vi "main.vi"() -> ()   [LabVIEW 2021]
uses:
  daq.ctl
  gpibusb.ctl
  calib.ctl
  <vilib>/Analysis/6fits.llb/Curve Fitting Criteria.ctl
  daq_FSM.vi
  Arduino_FlowPump_Controller.vi
  <vilib>/ErrorRing/Error Ring.xnode
  DAQ.lvlib
  CALIBRATION.lvlib
  statistics.lvlib
  <vilib>/Analysis/NI_AALPro.lvlib
  <vilib>/Analysis/NI_AALBase.lvlib
  GPIB_UART.lvlib
  Certification.lvlib
panel:
  out "Hysteresis Graph":cluster{dbl[], "Media":dbl[]}[](graph)
  out "Uncertainty linearity error":dbl
  out "Hysteresis Uncertainty":dbl
  out "Accuracy Reference Instrument (FS-2012)":dbl
  out "Standard Uncertainty DAQ (mL/min)":dbl
  out "sum of squared errors":dbl
  out "max value":dbl
  out "x/y":dbl
  out "Array":dbl[](array[numeric])
  out "Media 2":dbl[](array[numeric])
  out "Media":dbl[](array[numeric])
  out "Max Uncertainty\n (Descending) [mV]":dbl format="%_1f"
  out "Max Uncertainty\n (Ascending) [mV]":dbl format="%#_2f"
  out "Max Combined \nUncertainty (RSS) [mL/min]\n\n2":dbl format="%_3f"
  out "Max Uncertainty\n (Ascending) [mL/min]\n\n2":dbl format="%_3f"
  out "Max Uncertainty\n (Descending) [mL/min]\n\n2":dbl format="%_3f"
  out "Max Combined \nUncertainty (RSS) [mV]":dbl format="%.1f"
  out "digital_salita_2":dbl[][](array[numeric])
  out "digital_salita_1":dbl[][](array[numeric])
  out "digital_discesa_2":dbl[][](array[numeric])
  out "digital_discesa_1":dbl[][](array[numeric])
  out "analog_salita_2":dbl[][](array[numeric])
  out "analog_salita_1":dbl[][](array[numeric])
  out "analog_discesa_2":dbl[][](array[numeric])
  out "analog_discesa_1":dbl[][](array[numeric])
  out "Max Uncertainty Descending":dbl format="%#.1f"
  out "Max Uncertainty Asending.":dbl format="%#.1f"
  out "abs(x)":dbl[](array[numeric])
  out "difference":dbl[](array[numeric])
  out "asc_table":dbl[][](array[numeric])
  out "disc_table 2":dbl[][](array[numeric])
  out "Estimate Ascending":dbl[](array[numeric])
  out "Estimate Descending":dbl[](array[numeric])
  out "Best Linear Fit D2":dbl[](array[numeric])
  out "Best Linear Fit D":dbl[](array[numeric])
  out "total_flow":dbl[][](array[numeric])
  out "Best Linear Fit A":dbl[](array[numeric])
  out "Standard Uncertainty DAQ (mV)":dbl
  out "eqA":string
  out "eqD":string
  out "Table Strings":string[][](array[string])
  out "step_":i32
  out "start_":i32
  in  "scale_analog":dbl=1000.0
  in  "scale_digital":dbl=1000.0
  out "Input Sequence":dbl[](array[numeric])
  in  "Tab Control":T1(tab)
  in  "Tab Control 7":enum32{"POWER PANEL", "Contacts"}(tab)
  in  "POWER":bool=TRUE
  in  "POWER 2":bool=TRUE
  in  "POWER 3":bool=TRUE
  in  "Base Programs Path":path=path "C:/Users/anton/Desktop/mapi-master"
  out "String":string="Welcome! This is the main application to use in order to calibrate the analog flow sensor, Renesas FS-1012.\n\nThe picture to the left shows the instruments that you will need to connect to use this application. These are:\na) NI DAQ-6008 Data Acquisition Board\nb) Conditioning circuit\nc) Analog (under test) Flow Sensor, Renesas FS-1012\nd) Digital (reference) Flow Sensor, Renesas FS-2012\ne) air-pump\nf) Power Generator Agilent e36436A\ng) Power Supply QL355TP\n\n\nEach Tab in the application allows to perform the many steps that compose the calibration procedure to follow in order to be able to convert the raw output of the sensor (voltage, in mV) into a significant measure (flow, in liters-per-minute). \n\nThe following is a brief description of what each tab enables to accomplish:\n1) Acquisition: this tab enables you to perform acquisitions from both sensors as well as save the acquired samples in specified files.\n2) Datasets: this tab enables you to load the stored dataset to begin the analysis of each sensor.\n3) Visual Exploration: this tab enables you to get a first view of the statistical distribution of the samples in each dataset, through histograms and boxplots.\n4) Results: this tab is used to compare the measurements acquired during ascending and descending input sequences in order to verify the occurrence of the hysteresis phenomena. Also, sensor accuracy is reported in specified indicators.\n5) Comparison: this tab enable the user to compare the plot of ascending and descending curves of both sensors, in order to determine whether the measurements taken from the two instruments share some kind of correlation.\n6) Curve Fitting: this tab enables you to compute the best-fit equations to predict the output value of each sensor given the input current that drives the air-pump, which in turn generates an airflow measured by the two sensors, respectively.\n7) Instruments Control: this tab should be used only be expert users. It enables you to control directly the power generator and the Arduino UNO, through dedicated controls.\n\nReference manuals will explain in more detail the correct way to use this application!"
  in  "Tab Control 8":T2(tab)
  out "FS-2012 ON|OFF 2":bool
  out "POWER_SUPPLY ON|OFF 2":bool
  out "DAQ ON|OFF":bool
  out "FS-1012 ON|OFF":bool
  out "ARDUINO ON|OFF 2":bool
  in  "gpib address":string(combo)="1"
  in  "serial port":string(combo)="COM5"
  in  "Channel":string(combo)="Dev1/ai0"
  in  "Phase":string(combo)="tabella_salita"
  in  "Ring 2":u16(ring)=1 items=["Dataset 1"=1, "Dataset 2"=2]
  in  "Read":bool
  in  "Samples":i32=100
  in  "Control Panel":T3={"Enable"=FALSE, "Step [mA]"=0, "Next"=FALSE, "Start [mA]"=400} {"Start [mA]" min=0 max=1000 step=25; "Step [mA]" min=0 max=1000 step=25}
  out "output current":i32(knob)=400 scale=0.0..700.0
  in  "Dataset A Path":path=path "C:/Users/anton/Desktop/Measurements_stuff/sandbox/last"
  in  "Dataset D Digital":path=path "C:/Users/anton/Desktop/Measurements_stuff/sandbox/last"
  in  "Tab Control 2":enum32{"Live Acquisition", "Datasets"}(tab)
  out "volt":dbl format="%#_3g"
  out "flow":dbl
  in  "Buffer Size (Sa)":string(combo)="1000"
  in  "Sampling Rate (Sa/s)":string(combo)="1000"
  in  "Scale Voltage":string(combo)="(mV)"
  in  "Sampling Frequency (Hz)":string(combo)="1.5"
  in  "Scale Flow":string(combo)="(mL/min)"
  out "Analog  Flow Sensor":dbl[](graph)
  out "Digital  Flow Sensor":dbl[](graph)
  in  "DATASET_CLEAR":bool
  in  "DATASET_STORE":bool
  out "Flow Rate (mL/min)":dbl[](array[numeric])
  out "Voltage (mV)":dbl[](array[numeric]) format="%#_3g"
  out "Analog Dataset":dbl[][](array[numeric]) format="%#_3g"
  out "Digital Dataset":dbl[][](array[numeric]) format="%#.3g"
  in  "Save":bool
  in  "Plot Signals":bool
  out "Features":i32
  out "tot_samples":i32
  in  "Up Button 2":bool
  in  "Up Button":bool
  in  "Analog_salita2":path=path "C:/Users/anton/Desktop/mapi-master/misure_17_10_A/tab_salita2.csv"
  in  "Analog_salita1":path=path "C:/Users/anton/Desktop/mapi-master/misure_17_10_A/tab_salita1.csv"
  in  "Analog_discesa2":path=path "C:/Users/anton/Desktop/mapi-master/misure_17_10_A/tab_discesa2.csv"
  in  "Analog_discesa1":path=path "C:/Users/anton/Desktop/mapi-master/misure_17_10_A/tab_discesa1.csv"
  in  "Digital_discesa2":path=path "C:/Users/anton/Desktop/mapi-master/misure_17_10_D/tab_discesa2.csv"
  in  "Digital_discesa1":path=path "C:/Users/anton/Desktop/mapi-master/misure_17_10_D/tab_discesa1.csv"
  in  "CLEAR BUTTON":bool
  in  "Load Files":bool
  in  "?":enum32{"FS-1012 A", "FS-1012 D"}(tab)
  out "Analog Salita":dbl[][](array[numeric])
  out "Analog Discesa":dbl[][](array[numeric])
  in  "Digital_salita2":path=path "C:/Users/anton/Desktop/mapi-master/misure_17_10_D/tab_salita2.csv"
  in  "Digital_salita1":path=path "C:/Users/anton/Desktop/mapi-master/misure_17_10_D/tab_salita1.csv"
  in  "?":enum32{"FS-2012 D", "FS-2012 A"}(tab)
  out "Digital Discesa":dbl[][](array[numeric])
  out "Digital Salita":dbl[][](array[numeric])
  out "L1":dbl format="%.1f"
  out "U1":dbl format="%.1f"
  in  "index":string(combo)="12" caption="Input Current (mA)"
  in  "Ring":u16(ring)=1 items=["Dataset 2", "Dataset 1"]
  in  "Histogram intervals":i32=10
  in  "Sensor & Phase":T4(ring)=enum."Analog (Decreasing Values)"
  in  "Tab Control 3":enum32{"Histogram", "Boxplot"}(tab)
  out "Histogram":cluster{"X Values":dbl[], dbl[]}[](graph)
  out "Box Plot":cluster{dbl[], dbl[]}[](graph)=[{[7.857142857142858, 2.142857142857143, 2.142857142857143, 7.857142857142858, 7.857142857142858, 2.142857142857143, 2.142857142857143], [0.6526, 0.6526, 0.6514, 0.6514, 0.6538, 0.6538, 0.6526]}, {[], []}, {[5.0, 5.0], [0.6489, 0.6569]}, {[5.0, 5.0], [0.6538, 0.6562000000000001]}, {[5.0, 5.0], [0.6514, 0.6489999999999998]}, {[6.428571428571429, 3.571428571428571], [0.6562000000000001, 0.6562000000000001]}, {[6.428571428571429, 3.571428571428571], [0.6489999999999998, 0.6489999999999998]}, {[17.857142857142858, 12.142857142857142, 12.142857142857142, 17.857142857142858, 17.857142857142858, 12.142857142857142, 12.142857142857142], [0.66495, 0.66495, 0.6635, 0.6635, 0.6662, 0.6662, 0.66495]}, {[15.0, 15.0], [0.6921, 0.6851]}, {[15.0, 15.0, 15.0, 15.0, 15.0, 15.0], [0.6591, 0.6608, 0.6604, 0.6607, 0.671, 0.6606]}, {[15.0, 15.0], [0.6662, 0.669]}, {[15.0, 15.0], [0.6635, 0.6609]}, {[16.428571428571427, 13.571428571428571], [0.669, 0.669]}, {[16.428571428571427, 13.571428571428571], [0.6609, 0.6609]}, {[27.857142857142858, 22.142857142857142, 22.142857142857142, 27.857142857142858, 27.857142857142858, 22.142857142857142, 22.142857142857142], [0.6796, 0.6796, 0.6789, 0.6789, 0.6803, 0.6803, 0.6796]}, {[], []}, {[25.0, 25.0, 25.0, 25.0, 25.0, 25.0, 25.0, 25.0, 25.0], [0.677, 0.6769, 0.6774, 0.6768, 0.6772, 0.6757, 0.6762, 0.6818, 0.6823]}, {[25.0, 25.0], [0.6803, 0.6817000000000001]}, {[25.0, 25.0], [0.6789, 0.6774999999999999]}, {[26.428571428571427, 23.571428571428573], [0.6817000000000001, 0.6817000000000001]}, {[26.428571428571427, 23.571428571428573], [0.6774999999999999, 0.6774999999999999]}]
  out "Q3":dbl format="%.1f"
  out "Q1":dbl format="%.1f"
  out "Mean":dbl format="%.2f"
  out "Standard Deviation":dbl format="%.2f"
  out "Median":dbl format="%.1f"
  in  "Tab Control 6":T5(tab)
  out "Ascending Table":dbl[][](array[numeric]) format="%#.1f"
  out "Descending Table":dbl[][](array[numeric]) format="%#.1f"
  out "uncda":dbl[](array[numeric]) caption="Type A Standard Uncertainties FS-2012 (mL/min)" format="%#.1f"
  out "Standard Deviations FS-1012 (mV)":dbl[](array[numeric]) format="%#_2f"
  out "Standard Deviations FS-2012 (mL/min)":dbl[](array[numeric]) format="%#.1f"
  out "Expected Values FS-1012 (mV)":dbl[](array[numeric]) format="%#.1f"
  out "Expected Values FS-2012 (mL/min)":dbl[](array[numeric]) format="%#.1f"
  out "uncaa":dbl[](array[numeric]) caption="Type A Standard Uncertainties FS-1012 (mV)" format="%#.1g"
  out "uncdd":dbl[](array[numeric]) caption="Type A Standard Uncertainties FS-2012 (mL/min)" format="%#.1f"
  out "uncad":dbl[](array[numeric]) caption="Type A Standard Uncertainties FS-1012 (mV)" format="%#.1f"
  out "stdad":dbl[](array[numeric]) caption="Standard Deviations FS-1012 (mV)" format="%#_2g"
  out "stddd":dbl[](array[numeric]) caption="Standard Deviations FS-2012 (mL/min)" format="%#.1f"
  out "exad":dbl[](array[numeric]) caption="Expected Values FS-1012 (mV)" format="%#.1f"
  out "exdd":dbl[](array[numeric]) caption="Expected Values FS-2012 (mL/min)" format="%#.1f"
  in  "Tab Control 5":T6(tab)
  out "COMPARISON":T7(graph)
  out "FS-1012 Ascending & Descending Curves":T8(graph)
  out "FS-2012 Ascending & Descending Curves":T8(graph)
  in  "Tab Control 9":T9(tab)
  out "A":cluster{"Media":dbl[], "Media":dbl[]}[](graph) caption="FS-1012 Ascending & Descending Curves"
  out "A 2":cluster{"Media":dbl[], dbl[]}[](graph) caption="FS-1012 Ascending & Descending Curves"
  out "D":cluster{"Media":dbl[], "Media":dbl[]}[](graph) caption="FS-1012 Ascending & Descending Curves"
  out "D 2":cluster{"Media":dbl[], dbl[]}[](graph) caption="FS-1012 Ascending & Descending Curves"
  in  "Tab Control 4":enum32{"Regression", "Linearization"}(tab)
  out "RMSE 2":dbl format="%#.1f"
  out "R_sqr":dbl format="%#_3g"
  out "m":dbl format="%#.2f"
  out "b":dbl format="%#.1f"
  out "Calibration Conversion Equation":string="V = m·F + b"
  out "Ascending Table 2":dbl[][](array[numeric]) format="%#.1f"
  out "nonlinearity":dbl format="%#.2f"
  in  "Plot":enum32{"Item 0", "Radio Selection 4"}(radio)=enum."Radio Selection 4"
  out "Calibration Curve":cluster{dbl[], "Media":dbl[]}[](graph)
  in  "Tab Control 10":enum32{"Calibration Curve", "Accuracy"}(tab)
  out "R-square avg":dbl format="%#.2f"
  out "RMSE_avg":dbl format="%#.2f"
  out "b avg":dbl format="%#.1f"
  out "m avg":dbl format="%#.2f"
  out "Calibration Conversion Equation 2":string="V = m·F + b"
  out "Absolute Uncertainty in %FSO":dbl format="%#.2f"
  out "Expanded Uncertainty in %FSO":dbl format="%#.2f"
  out "Nonlinearity %FSO":dbl format="%#.2f"
  out "Hysteresis %FSO":dbl format="%#.2f"
  out "Max Uncertainty":dbl format="%#.1f"
  out "Max Deviation":dbl format="%#.1f"
  out "Absolute Uncertainty":dbl format="%#.1f"
  out "Expanded Uncertainty":dbl format="%#.1f"
  in  "calibrate!":bool
  in  "Arduino":string="Arduino UNO R3"
  in  "Air Pump":string="EAD NEO PP2"
  in  "DAQ":string="NI USB-6008"
  in  "PSU A":string="Agilent, Type e3634A"
  in  "Gas used":string="Air"
  in  "DAQ Resolution":string="4,88"
  in  "Location":string="PalaUnisannio"
  in  "Manufacturer":string="Renesas Electronic Company"
  in  "Operator":string="User1"
  in  "Date":string="28/07/2025"
  in  "Temperature":string="25°C"
  in  "Sensing Range":string="0 -10 L/m"
  in  "Series":string="FS-1012-1100-NG"
  in  "Description":string="Gas Flow Meter"
  # "Max Uncertainty\nAscending"
  # "(mL/min)"
  # "(mL/min)"
  # "Max Uncertainty\nDescending"
  # "(mL/min)"
  # "Offset"
  # "Max [mL/min]"
  # "QUICK GUIDE"
  # "DAQ"
  # "MAIN"
  # "GPIB_USB"
  # "mapiflowproject@gmail.com"
  # "programmable power generator"
  # "NI DAQ\nUSB-6008"
  # "ArduinoUNO"
  # "Air-pump"
  # "external \n  power \n  generator"
  # "FS-2012"
  # "FS-1012"
  # "conditioning_circuit"
  # "MEASUREMENT SYSTEM SETUP"
  # "ARDUINO & POWER SUPPLY"
  # "NI-DAQ USB 6008"
  # "ACQUISITION"
  # "Control Panel"
  # "Air Pump\nCurrent [mA]"
  # "FS-2012"
  # "Flow"
  # "FS-1012"
  # "Voltage"
  # "FS-1012"
  # "FS-2012"
  # "D"
  # "A"
  # "DATASETS"
  # "FS-1012"
  # "FS-2012"
  # "Descending Phase"
  # "Descending Phase"
  # "DATASET 1"
  # "DATASET 1"
  # "DATASET 2"
  # "DATASET 2"
  # "Ascending Phase"
  # "DATASET 1"
  # "DATASET 2"
  # "Features Found"
  # "Total No. of Samples"
  # "Analog Sensor Files Here!"
  # "Digital Sensor Files Here!"
  # "(mV)"
  # "Ascending Phase"
  # "(mV)"
  # "Descending Phase"
  # "Ascending Phase"
  # "DATASET 1"
  # "DATASET 2"
  # "(mL/min)"
  # "Descending Phase"
  # "Descending Phase"
  # "(mL/min)"
  # "Ascending Phase"
  # "SETTINGS"
  # "HISTOGRAM"
  # "Mean"
  # "Standard Deviation"
  # "BOXPLOT"
  # "Lower Whisker"
  # "Lower Quartile"
  # "Upper Whisker"
  # "Upper Quartile"
  # "Median"
  # "VISUALIZE"
  # "RESULTS"
  # "Ascending Phase"
  # "FS-1012 (mV)                     | FS-2012 (mL/min)"
  # "Descending Phase"
  # "FS-1012 (mV)                    | FS-2012 (mL/min)"
  # "Comparison Graph"
  # "Ascending Phase Curve"
  # "Descending Phase Curve"
  # "BEST LINEAR FIT"
  # "LINEAR REGRESSION Curve"
  # "Estimated Flow vs. Calibrated Reference"
  # "LINEAR REGRESSION Curve"
  # "Estimated Flow vs. Calibrated Reference"
  # "("
  # ")"
  # "mV"
  # "m"
  # "________"
  # "(mV)"
  # "RMSE"
  # "mL/min"
  # "b"
  # "2"
  # "R"
  # "(mV)"
  # "Linear Regression Equation"
  # "Nonlinearity (%FSO)"
  # "Reference [mL/min]    | DUT       [mL/min]     | Deviation [mL/min]"
  # "Calibration Curve"
  # "Calibration Function f(F)"
  # "("
  # ")"
  # "mV"
  # "m"
  # "b"
  # "________"
  # "(mV)"
  # "mL/min"
  # "2"
  # "R"
  # "RMSE (mV)"
  # "Max. Deviation\n(Asc. vs. Desc.)"
  # "(mL/min)"
  # "Hysteresis"
  # "(%FSO)"
  # "Ascending, Descending Phase\nCombined  Uncertainty (RSS)"
  # "Nonlinearity"
  # "(%FSO)"
  # "(mL/min)"
  # "Measuring System \nAbsolute Uncertainty (%FSO)"
  # "Measuring System \nCombined Uncertainty (mL/min)"
  # "Expanded  Absolute Uncertainty, k = 2  (%FSO)"
  # "Expanded  Combined Uncertainty, k = 2  (mL/min)"
  # "Manufacturer"
  # "Description"
  # "Gas Used"
  # "PSU"
  # "Sensing Range (Nominal)"
  # "Series"
  # "DAQ Resolution (mV)"
  # "DAQ"
  # "Flow Pump"
  # "Arduino"
  # "Environment Temperature"
  # "Date"
  # "Operator"
  # "Location"
  # "Instrumentation Used"
  # "General Informations"
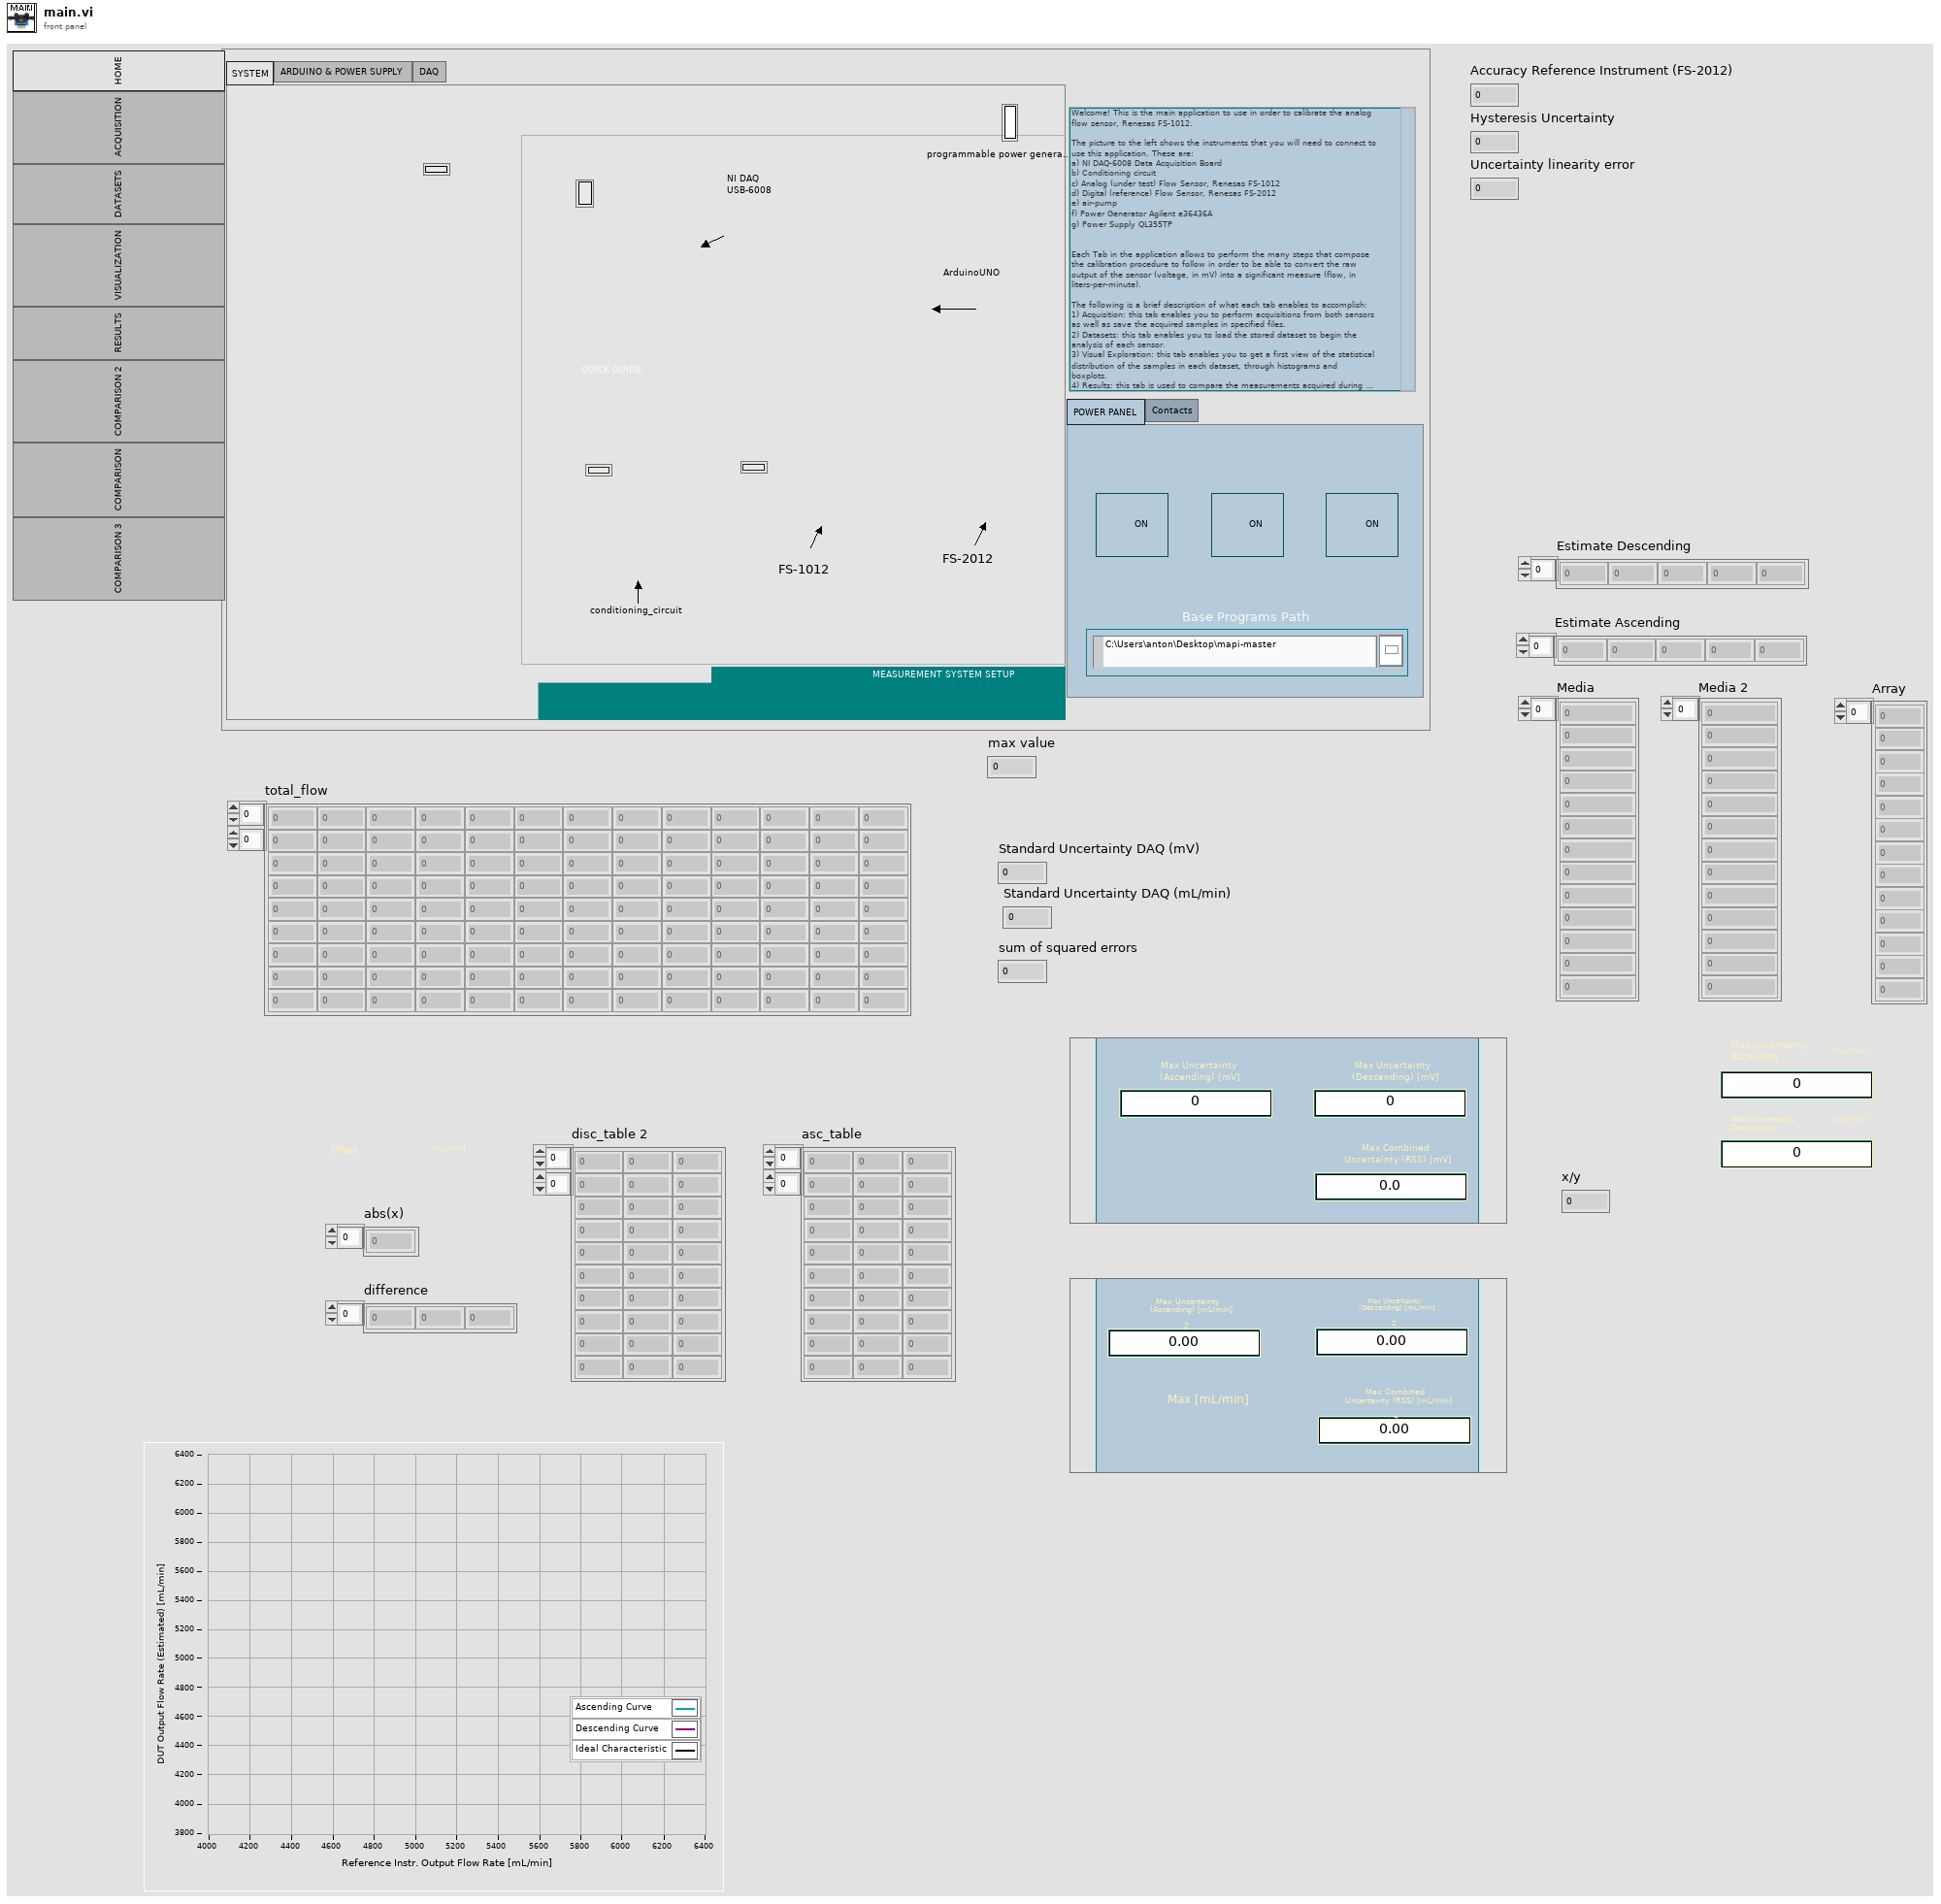
[diagram p1: front panel]
types:
  T1 = enum32{"HOME", "ACQUISITION", "DATASETS", "VISUALIZATION", "RESULTS", "COMPARISON 2", "COMPARISON", "COMPARISON 3"}
  T2 = enum32{"SYSTEM", "ARDUINO & POWER SUPPLY", "DAQ"}
  T3 = cluster{"Enable":bool, "Step [mA]":i32, "Next":bool, "Start [mA]":i32}
  T4 = enum16{"Analog (Increasing Values)", "Analog (Decreasing Values)", "Digital (Decreasing Values)", "Digital (Increasing Values)"}
  T5 = enum32{"Comparison Tables", "Analysis (A)", "Analysis (D)"}
  T6 = enum32{"Comparison", " Ascending", " Descending"}
  T7 = cluster{"Array":dbl[], "media_combinata":dbl[]}[]
  T8 = cluster{"media_combinata":dbl[], "Array":dbl[]}[]
  T9 = enum32{"Ascending (Voltage vs. Flow)", "Ascending (Flow in vs. Flow Out)", "Descending (Voltage vs. Flow)", "Descending (Flow in vs. Flow out)"}
  T10 = typedef "calib.ctl" = enum16{"wait", "linearization", "certificate", "linear regression", "simulate", "results4", "result3", "curves", "fitting", "results2", "combined uncertainty", "results", "boxplot", "scatterplot", "comparison", "histogram", "error", "curve_fitting", "calibration curve", "uncertainty", "load_measures", ""}
  T11 = typedef "gpibusb.ctl" = enum16{"INIT", "FREQ", "CURR?", "CURR", "READ_DIGITAL", "START", "STOP", "ACQUIRE", "STEP", "ARDUINO_SETTINGS", "NEXT", "SHUTDOWN", "ERROR"}
  T12 = typedef "daq.ctl" = enum16{"INIT", "PARAMETERS", "READ", "READ_VOLTAGE", "STOP", "DAQ_SETTINGS", "ERROR", "FLUSH", "SHUTDOWN", "CLEAR"}
  T13 = enum8{"Enabled", "Disabled", "Disabled and Grayed Out"}
  T14 = cluster{"Description":string, "Manufacturer":string, "Series":string, "Sensing Range":string, "Operator":string, "Temperature":string, "PSU A":string, "PSU B":string, "Gas used":string, "Air Pump":string, "DAQ":string, "Arduino":string}
  T15 = typedef "NI_AALPro.lvlib/Curve Fitting Criteria.ctl" = u16
  T16 = cluster{"Media":dbl[], "Best Linear Fit":dbl[]}[]
  T17 = cluster{"Media":dbl[], "Estimate Descending":dbl[]}
  T18 = cluster{"Media":dbl[], "Estimate Ascending":dbl[]}
  T19 = cluster{"Media":dbl[], "Estimate Ascending":dbl[]}[]
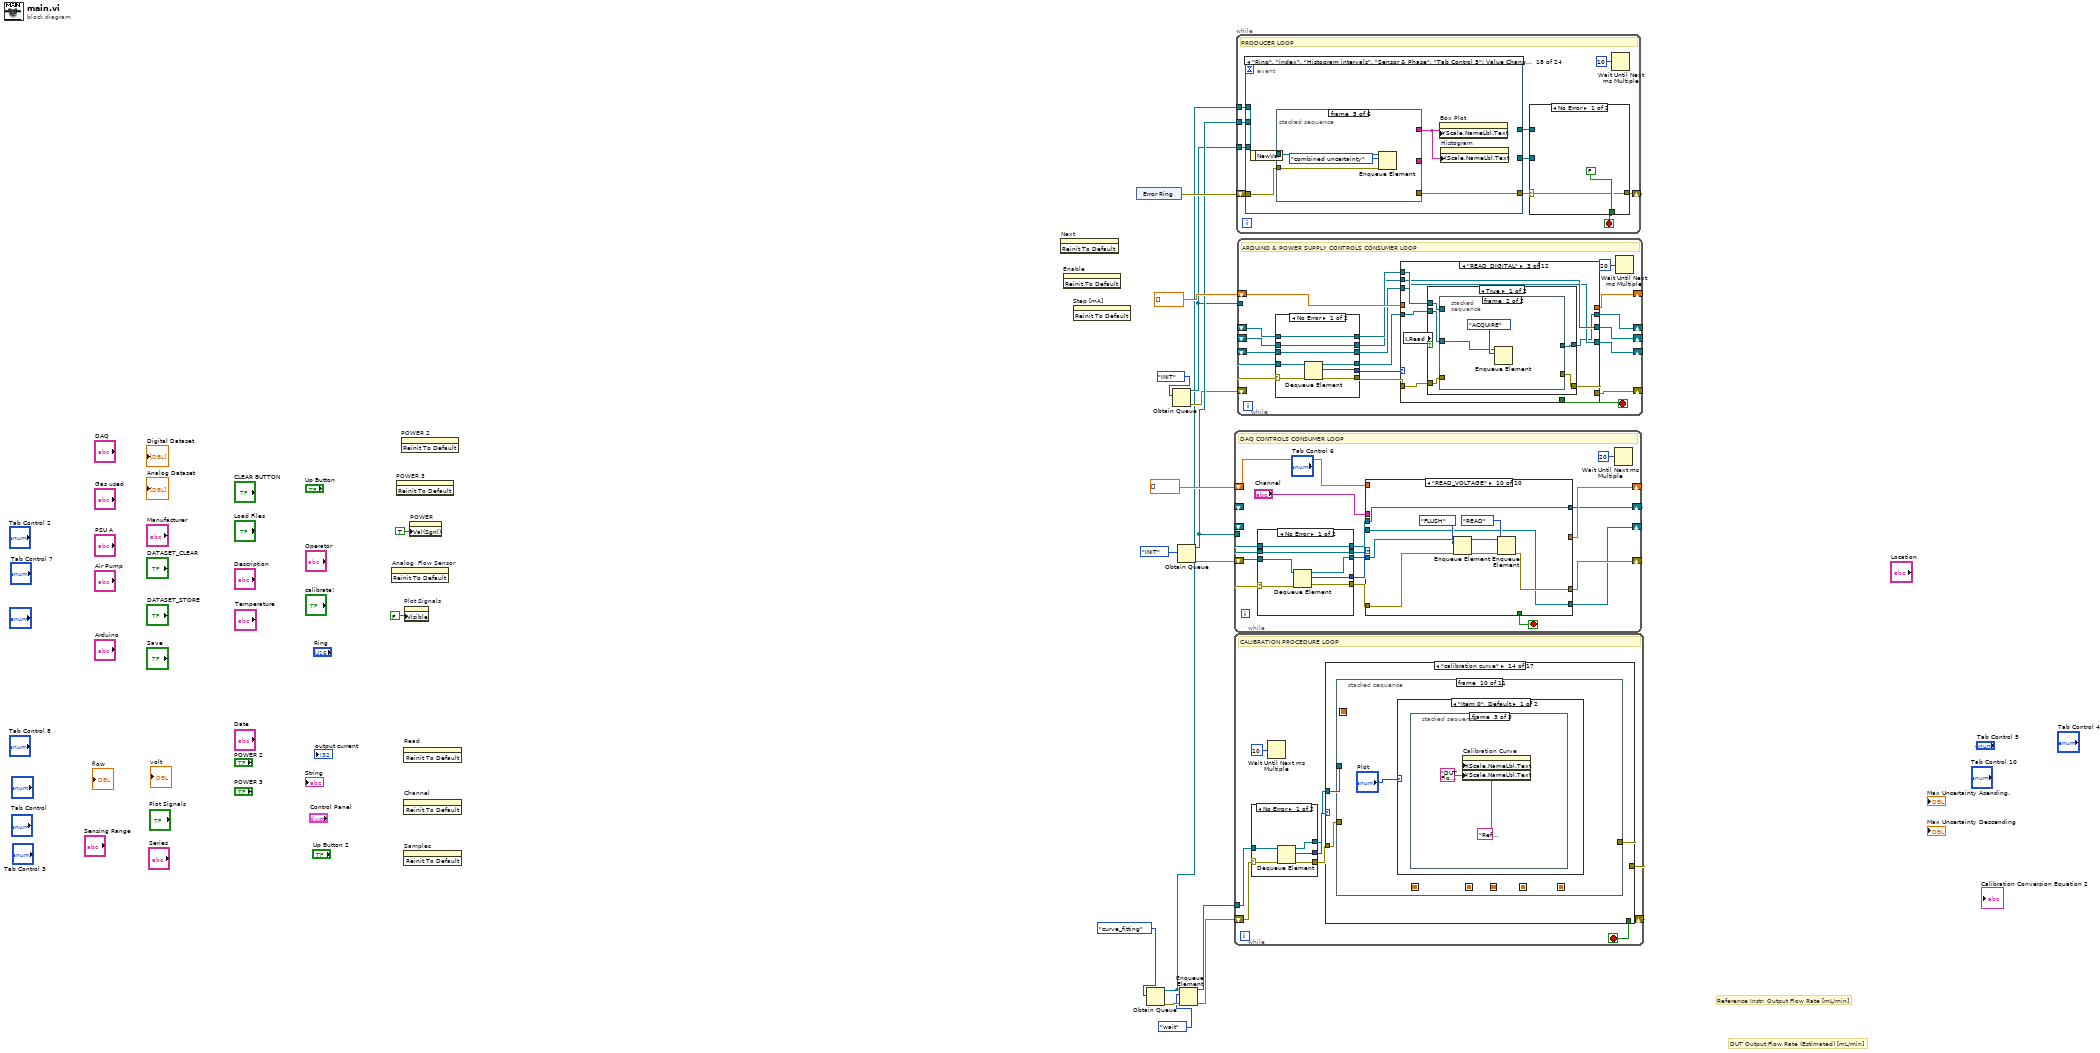
[diagram p0: block diagram]
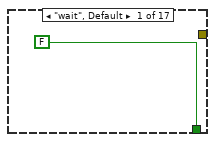
[diagram p2: hidden frame]
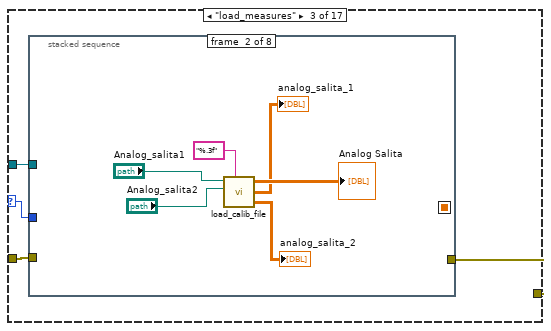
[diagram p4: hidden frame]
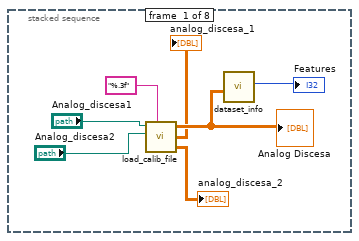
[diagram p5: hidden frame]
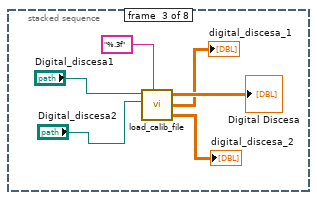
[diagram p6: hidden frame]
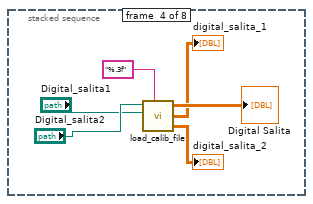
[diagram p7: hidden frame]
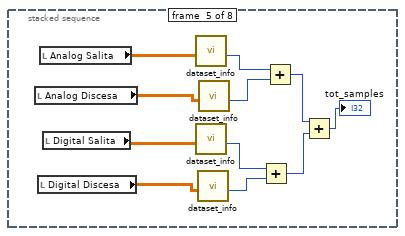
[diagram p8: hidden frame]
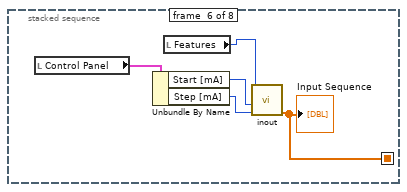
[diagram p9: hidden frame]
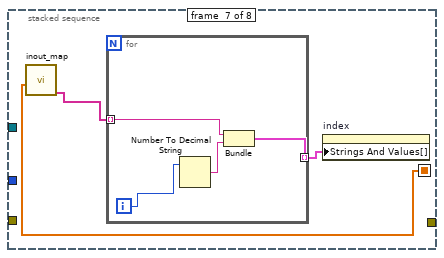
[diagram p10: hidden frame]
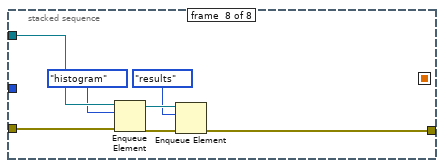
[diagram p11: hidden frame]
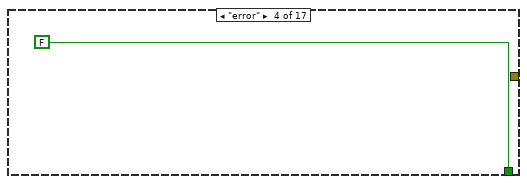
[diagram p12: hidden frame]
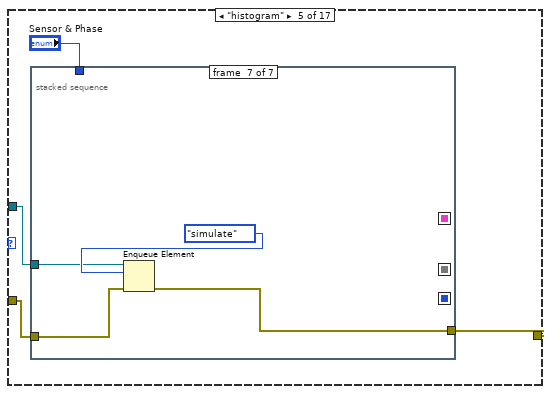
[diagram p13: hidden frame]
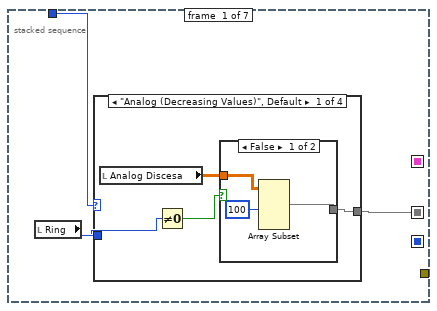
[diagram p14: hidden frame]
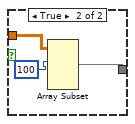
[diagram p15: hidden frame]
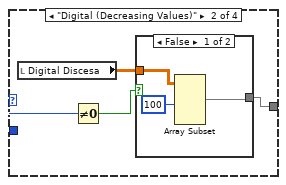
[diagram p16: hidden frame]
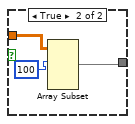
[diagram p17: hidden frame]
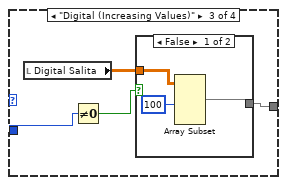
[diagram p18: hidden frame]
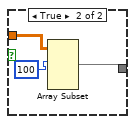
[diagram p19: hidden frame]
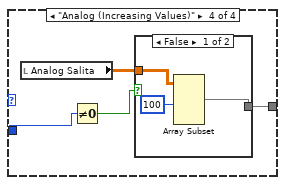
[diagram p20: hidden frame]
diagram:
  # "DUT Output Flow Rate (Estimated) [mL/min]"
  # "Reference Instr. Output Flow Rate [mL/min]"
  n1 = invoke on="Analog  Flow Sensor" class="WFGraph (strict)" method="Reinit To Default"() -> ()  [unwired: 3 in, 3 out]
  n2 = invoke on="POWER 3" class="Bool (strict)" method="Reinit To Default"() -> ()  [unwired: 3 in, 3 out]
  n3 = invoke on="POWER 2" class="Bool (strict)" method="Reinit To Default"() -> ()  [unwired: 3 in, 3 out]
  n4 = invoke on="Read" class="Bool (strict)" method="Reinit To Default"() -> ()  [unwired: 3 in, 3 out]
  n5 = invoke on="Channel" class="CmbBox" method="Reinit To Default"() -> ()  [unwired: 3 in, 3 out]
  n6 = invoke on="Samples" class="DigNum (strict)" method="Reinit To Default"() -> ()  [unwired: 3 in, 3 out]
  n7 = property on="Plot Signals" class="Bool"("Visible"=FALSE) -> ()  [unwired: 2 in, 2 out]
  n8 = property on="POWER" class="Bool (strict)"("Val(Sgnl)"=TRUE ("Value (Signaling)")) -> ()  [unwired: 2 in, 2 out]
  n9 = invoke on="Next" class="Bool (strict)" method="Reinit To Default"() -> ()  [unwired: 3 in, 3 out]
  n10 = invoke on="Enable" class="Bool (strict)" method="Reinit To Default"() -> ()  [unwired: 3 in, 3 out]
  n11 = invoke on="Step [mA]" class="DigNum (strict)" method="Reinit To Default"() -> ()  [unwired: 3 in, 3 out]
  n12 = xnode "Error Ring"() -> ("error out"=w14:errorcluster)
  n13 = Obtain Queue(element data type=calib."curve_fitting" ("Enum")) -> (queue out=w2:refnum<queue>, error out=w6:errorcluster)  [unwired: 4 in, 1 out]
  n14 = Obtain Queue(element data type=gpibusb."INIT" ("element")) -> (queue out=w10:refnum<queue>, error out=w9:errorcluster)  [unwired: 4 in, 1 out]
  n15 = Obtain Queue(element data type=daq."INIT" ("STATE")) -> (queue out=w11:refnum<queue>, error out=w8:errorcluster)  [unwired: 4 in, 1 out]
  n16 = Enqueue Element(queue=w2, element=calib."wait", error in (no error)=w6) -> (queue out=w4:refnum<queue>, error out=w5:errorcluster)  [unwired: 1 in, 1 out]
  n17 = while {
    tunnel: w11 -> [w33]
    shift-right: [w27] -> _
    shift-left: dbl[] [] -> [w28]
    shift-right: [w26] -> _
    shift-left: w8 -> [w34]
    shift-right: [w24] -> _
    shift-left: _ -> [w22]
    shift-right: [w23] -> _
    shift-left: _ -> [w21]
    stop <- w29 stop-if-true
    # "DAQ CONTROLS CONSUMER LOOP"
    n18 = case shown="No Error" w34 {
      selector: w34 -> [w40 w46]
      tunnel: w33 -> [w41 w44]
      tunnel: [w39 daq."ERROR" ("STATE")] -> w32
      tunnel: [w38 w46] -> w31
      tunnel: [w37 w44] -> w30
      tunnel: [w36 w43] -> w19
      tunnel: w22 -> [w36 w43]
      tunnel: [w35 w42] -> w20
      tunnel: w21 -> [w35 w42]
      frame No Error {
        n19 = Dequeue Element(queue=w41, error in (no error)=w40) -> (queue out=w37:refnum<queue>, element=w39:T12, error out=w38:errorcluster)  [unwired: 1 in, 1 out]
      }
      frame Error {
      }
    }
    n20 = case shown="\"READ_VOLTAGE\"" w32 {
      tunnel: w31 -> [w51 w56 w88 w129 w136 w139 w156 w162 w169 w177]
      tunnel: w30 -> [w52 _ w87 _ _ _ _ _ _ w181]
      tunnel: [FALSE FALSE _ _ _ _ _ _ _ _] -> w29
      tunnel: w28 -> [_ _ w90 _ _ _ _ _ _ _]
      tunnel: [_ _ w85 _ _ _ _ _ _ _] -> w27
      tunnel: [w49 w55 w86 w128 _ _ _ w166 w168 w175] -> w26
      tunnel: "Channel" -> [_ _ _ _ w134 _ _ _ _ _]
      tunnel: [w48 w54 w91 w125 w131 w138 w159 w164 w172 w174] -> w24
      tunnel: [w47 w53 w84 w126 w130 w137 w158 w165 w171 w173] -> w23
      tunnel: w20 -> [w47 _ w89 w127 w130 w137 w158 w165 w171 w173]
      tunnel: w19 -> [w48 _ w91 w125 w132 w140 w159 w163 w172 w174]
      frame "ERROR" {
        n21 = Release Queue(queue=w52, error in (no error)=w51) -> (error out=w49:errorcluster)  [unwired: 1 in, 2 out]
      }
      frame "INIT", Default {
        n22 = local read "Base Programs Path"() -> (w57:path)
        n23 = stacked-sequence {
          seq-local: [w61 _ _ _ _ _ _ _ _] -> [_ _ _ _ w73 _ _ _ _]
          seq-local: [_ w64 _ _ _ _ _ _ _] -> [_ _ _ _ _ w76 _ _ _]
          seq-local: [_ _ w66 _ _ _ _ _ _] -> [_ _ _ _ _ w75 _ _ _]
          seq-local: [_ _ _ _ w72 _ _ _ _] -> [_ _ _ _ _ w80 w82 _ _]
          seq-local: [_ _ _ _ w69 _ _ _ _] -> [_ _ _ _ _ w79 _ _ _]
          seq-local: [_ _ _ _ _ w78 _ _ _] -> [_ _ _ _ _ _ _ _ _]
          tunnel: w56 -> [_ _ _ _ w71 _ w81 _ _]
          tunnel: w57 -> [w59 _ _ _ _ _ _ _ _]
          tunnel: [_ _ _ _ _ w76 _ _ _] -> w53
          tunnel: [_ _ _ _ _ _ w83 _ _] -> w55
          tunnel: [_ _ _ _ _ w75 _ _ _] -> w54
          frame #0 {
            # "compose program path"
            n24 = Path To String(path=w59) -> (string=w63:string)
            n25 = Concatenate Strings(w63, "\\labview\\daq_FSM.vi" ("string")) -> (w62:string)
            n26 = String To Path(string=w62) -> (path=w61:path)
          }
          frame #1 {
            n27 = Obtain Queue(element data type="") -> (queue out=w64:refnum<queue>)  [unwired: 4 in, 2 out]
          }
          frame #2 {
            n28 = Obtain Queue(element data type="") -> (queue out=w66:refnum<queue>)  [unwired: 4 in, 2 out]
          }
          frame #3 {
            w68 = TRUE ("Boolean 2")
            "DAQ ON|OFF" <- w68
            "FS-1012 ON|OFF" <- w68
          }
          frame #4 {
            n29 = vi-ref "DAQ.lvlib:daq_FSM.vi"() -> (w70:refnum<vi>)
            n30 = Open VI Reference(type specifier VI Refnum (for type only)=w70, vi path=w73, options=128, error in (no error)=w71) -> (vi reference=w72:refnum<vi>, error out=w69:errorcluster)  [unwired: 2 in]
          }
          frame #5 {
            n31 = call-by-ref "Start Asynchronous Call"(reference=w80, error in=w79, "loop rate"=u32 1000, "commands"=w75, "measurements"=w76) -> (error out=w78:errorcluster)  [unwired: 9 in, 1 out]
          }
          frame #6 {
            n32 = invoke on="DAQ CONTROL PANEL" class="SubPnl" method="Insert VI"(error in=w81, "VI Ref"=w82) -> (error out=w83:errorcluster)  [unwired: 2 in, 3 out]
          }
          frame #7 {
          }
          frame #8 {
          }
        }
      }
      frame "READ" {
        n33 = stacked-sequence {
          seq-local: [w97 _ _] -> [_ w102 w103]
          tunnel: w90 -> [w101 _ _]
          tunnel: w89 -> [w99 _ _]
          tunnel: w88 -> [w98 _ w105]
          tunnel: w87 -> [_ _ w106]
          tunnel: [_ w102 _] -> w85
          tunnel: [_ _ w104] -> w86
          tunnel: [w95 _ _] -> w84
          frame #0 {
            # "FETCH"
            n34 = Dequeue Element(queue=w99, error in (no error)=w98) -> (queue out=w95:refnum<queue>, element=w100:string)  [unwired: 1 in, 2 out]
            n35 = Fract/Exp String To Number(use system decimal point (T)=TRUE, string=w100) -> (number=w93:dbl)  [unwired: 2 in, 1 out]
            n36 = Multiply(x=w93, y="scale_analog") -> (x*y=w92:dbl)
            n37 = Build Array (concatenate)(w101, w92) -> (w97:dbl[])
            n38 = local write "volt"(w92) -> ()
          }
          frame #1 {
            # "update indicators"
            "Analog  Flow Sensor" <- w102
            "Voltage (mV)" <- w102
          }
          frame #2 {
            n39 = local read "Read"() -> (w107:bool)
            n40 = case shown="True" w107 {
              tunnel: w106 -> [_ w112]
              tunnel: [w108 w111] -> w104
              tunnel: w105 -> [w108 w110]
              tunnel: w103 -> [_ w109]
              frame False {
              }
              frame True {
                n41 = stacked-sequence {
                  seq-local: [w114 _ _] -> [_ w120 _]
                  seq-local: [_ w117 _] -> [_ _ w124]
                  tunnel: w112 -> [_ _ w123]
                  tunnel: [_ _ w122] -> w111
                  tunnel: w110 -> [_ _ w121]
                  tunnel: w109 -> [w113 _ _]
                  frame #0 {
                    n42 = Array Size(array=w113) -> (size(s)=w116:i32)
                    n43 = Greater Or Equal?(x=w116, y="Samples") -> (x >= y?=w114:bool)
                  }
                  frame #1 {
                    n44 = Select(t=daq."STOP" ("element"), s=w120, f=daq."READ") -> (s? t:f=w117:T12)
                  }
                  frame #2 {
                    n45 = Enqueue Element(queue=w123, element=w124, error in (no error)=w121) -> (error out=w122:errorcluster)  [unwired: 1 in, 2 out]
                  }
                }
              }
            }
          }
        }
      }
      frame "FLUSH" {
        n46 = Flush Queue(queue=w127, error in (no error)=w129) -> (queue out=w126:refnum<queue>, error out=w128:errorcluster)  [unwired: 1 out]
      }
      frame "DAQ_SETTINGS" {
        n47 = call "conc_state_args.vi"("State"="CONF_CH", "Args"=w134) -> ("state_and_args"=w133:string)  [unwired: 13 in]
        n48 = Enqueue Element(queue=w132, element=w133, error in (no error)=w136) -> (queue out=w131:refnum<queue>)  [unwired: 1 in, 2 out]
      }
      frame "PARAMETERS" {
        n49 = stacked-sequence {
          seq-local: [w143 _] -> [_ w151]
          seq-local: [w142 _] -> [_ w149]
          tunnel: w140 -> [w144 _]
          tunnel: [_ w150] -> w138
          tunnel: [_ w148] -> _
          tunnel: w139 -> [w141 _]
          frame #0 {
            n50 = call "conc_state_args.vi"("State"="CONF:PHY", "Args"="Sampling Rate (Sa/s)") -> ("state_and_args"=w145:string)  [unwired: 13 in]
            n51 = Enqueue Element At Opposite End(queue=w144, element=w145, error in (no error)=w141) -> (queue out=w143:refnum<queue>, error out=w142:errorcluster)  [unwired: 1 in, 1 out]
          }
          frame #1 {
            n52 = call "conc_state_args.vi"("State"="CONF:SAMPLES", "Args"="Buffer Size (Sa)") -> ("state_and_args"=w152:string)  [unwired: 13 in]
            n53 = Enqueue Element At Opposite End(queue=w151, element=w152, error in (no error)=w149) -> (queue out=w150:refnum<queue>, error out=w148:errorcluster)  [unwired: 1 in, 1 out]
          }
        }
      }
      frame "STOP" {
        n54 = property on="Read" class="Bool (strict)"(error in=w156, "Val(Sgnl)"=FALSE ("Value (Signaling)")) -> (error out=w155:errorcluster)  [unwired: 1 in, 1 out]
        n55 = property on="Samples" class="DigNum (strict)"(error in=w155, "DisabledEnum"=T13."Enabled" ("Disabled")) -> ()  [unwired: 1 in, 2 out]
      }
      frame "SHUTDOWN" {
        w161 = FALSE ("DAQ ON|OFF")
        n56 = local write "FS-1012 ON|OFF"(w161) -> ()
        n57 = local write "DAQ ON|OFF"(w161) -> ()
        n58 = Enqueue Element(queue=w163, element="SHUTDOWN", error in (no error)=w162) -> (queue out=w164:refnum<queue>, error out=w166:errorcluster)  [unwired: 1 in, 1 out]
      }
      frame "CLEAR" {
        n59 = property on="Samples" class="DigNum (strict)"(error in=w169, "DisabledEnum"=T13."Enabled" ("Disabled")) -> (error out=w168:errorcluster)  [unwired: 1 in, 1 out]
      }
      frame "READ_VOLTAGE" {
        n60 = Enqueue Element(queue=w181, element=daq."FLUSH", error in (no error)=w177) -> (queue out=w179:refnum<queue>, error out=w178:errorcluster)  [unwired: 1 in, 1 out]
        n61 = Enqueue Element(queue=w179, element=daq."READ", error in (no error)=w178) -> (error out=w175:errorcluster)  [unwired: 1 in, 2 out]
      }
    }
    n62 = Wait Until Next ms Multiple(millisecond multiple=u32 20) -> ()  [unwired: 1 out]
  }
  n63 = while {
    tunnel: w4 -> [w188]
    shift-right: [w182] -> _
    shift-left: w5 -> [w189]
    stop <- w186 stop-if-true
    # "CALIBRATION PROCEDURE LOOP"
    n64 = case shown="No Error" w189 {
      selector: w189 -> [w907 w910]
      tunnel: [w908 w910] -> w183
      tunnel: w188 -> [w906 w909]
      tunnel: [w905 calib."error" ("element")] -> w187
      tunnel: [w904 w909] -> w185
      frame No Error {
        n65 = Dequeue Element(queue=w906, error in (no error)=w907) -> (queue out=w904:refnum<queue>, element=w905:T10, error out=w908:errorcluster)  [unwired: 1 in, 1 out]
      }
      frame Error {
      }
    }
    n66 = Wait Until Next ms Multiple(millisecond multiple=u32 10) -> ()  [unwired: 1 out]
    n67 = case shown="\"calibration curve\"" w187 {
      selector: w187 -> [_ _ w193 _ _ _ _ _ _ _ _ _ _ _ _ _ _]
      tunnel: [FALSE _ _ FALSE _ _ _ _ _ _ _ _ _ _ _ _ _] -> w186
      tunnel: w185 -> [_ _ w194 _ w253 w337 w374 w380 w411 _ w432 w460 w534 w611 _ _ _]
      tunnel: w183 -> [_ _ w192 _ w254 w336 w373 w379 w410 _ w431 w459 w533 w610 _ _ _]
      tunnel: [_ _ w191 _ w251 w335 w371 w378 w409 _ _ w458 w532 w609 _ _ _] -> w182
      frame "wait", Default {
      }
      frame "boxplot" {
      }
      frame "load_measures" {
        n68 = stacked-sequence {
          seq-local: [_ _ _ _ _ w231 _ _] -> [_ _ _ _ _ _ w236 _]
          tunnel: w194 -> [_ _ _ _ _ _ _ w249]
          tunnel: w193 -> [_ _ _ _ _ _ _ _]
          tunnel: w192 -> [_ _ _ _ _ _ _ w247]
          tunnel: [_ _ _ _ _ _ _ w243] -> w191
          frame #0 {
            n69 = call "load_calib_file.vi"("file_1"="Analog_discesa1", "file_2"="Analog_discesa2", "format (%.3f)"="%.3f") -> ("insieme"=w197:dbl[][], "dataset1"=→"analog_discesa_1":dbl[][], "dataset2"=→"analog_discesa_2":dbl[][])  [unwired: 2 in]
            "Analog Discesa" <- w197
            n70 = call "dataset_info.vi"("Analog Salita"=w197) -> ("features"=→"Features":i32)  [unwired: 7 in, 3 out]
          }
          frame #1 {
            n71 = call "load_calib_file.vi"("file_1"="Analog_salita1", "file_2"="Analog_salita2", "format (%.3f)"="%.3f") -> ("insieme"=→"Analog Salita":dbl[][], "dataset1"=→"analog_salita_1":dbl[][], "dataset2"=→"analog_salita_2":dbl[][])  [unwired: 2 in]
          }
          frame #2 {
            n72 = call "load_calib_file.vi"("file_1"="Digital_discesa1", "file_2"="Digital_discesa2", "format (%.3f)"="%.3f") -> ("insieme"=→"Digital Discesa":dbl[][], "dataset1"=→"digital_discesa_1":dbl[][], "dataset2"=→"digital_discesa_2":dbl[][])  [unwired: 2 in]
          }
          frame #3 {
            n73 = call "load_calib_file.vi"("file_1"="Digital_salita2", "file_2"="Digital_salita1", "format (%.3f)"="%.3f") -> ("insieme"=→"Digital Salita":dbl[][], "dataset1"=→"digital_salita_1":dbl[][], "dataset2"=→"digital_salita_2":dbl[][])  [unwired: 2 in]
          }
          frame #4 {
            n74 = local read "Analog Discesa"() -> (w229:dbl[][])
            n75 = local read "Digital Discesa"() -> (w227:dbl[][])
            n76 = local read "Analog Salita"() -> (w230:dbl[][])
            n77 = local read "Digital Salita"() -> (w228:dbl[][])
            n78 = call "dataset_info.vi"("Analog Salita"=w230) -> ("samples"=w226:i32)  [unwired: 7 in, 3 out]
            n79 = call "dataset_info.vi"("Analog Salita"=w228) -> ("samples"=w224:i32)  [unwired: 7 in, 3 out]
            n80 = call "dataset_info.vi"("Analog Salita"=w227) -> ("samples"=w223:i32)  [unwired: 7 in, 3 out]
            n81 = call "dataset_info.vi"("Analog Salita"=w229) -> ("samples"=w225:i32)  [unwired: 7 in, 3 out]
            n82 = Add(x=w224, y=w223) -> (x+y=w221:i32)
            n83 = Add(x=w226, y=w225) -> (x+y=w222:i32)
            n84 = Add(x=w222, y=w221) -> (x+y=→"tot_samples":i32)
          }
          frame #5 {
            n85 = local read "Control Panel"() -> (w233:T3)
            n86 = Unbundle By Name(w233) -> ("Start [mA]"=w235:i32, "Step [mA]"=w234:i32)
            n87 = local read "Features"() -> (w232:i32)
            n88 = call "inout.vi"("Step [mA]"=w234, "Initial Value [mA]"=w235, "# Steps"=w232) -> ("Array"=w231:dbl[])  [unwired: 8 in]
            "Input Sequence" <- w231
          }
          frame #6 {
            n89 = call "inout_map.vi"("Input Sequence"=w236) -> ("array"=w237:string[])  [unwired: 10 in]
            n90 = for {
              tunnel: w237 -> [w242] mode=indexing
              tunnel: [w239] -> w238 mode=indexing
              i -> [w241]
              n91 = Number To Decimal String(number=w241) -> (decimal integer string=w240:string)  [unwired: 1 in]
              n92 = Bundle("format string"=w242, w240) -> (w239:cluster{"format string":string, string})  [unwired: 1 in]
            }
            n93 = property on="index" class="CmbBox"("Strings And Values[]"=w238) -> ()  [unwired: 2 in, 2 out]
          }
          frame #7 {
            n94 = Enqueue Element(queue=w249, element=calib."histogram", error in (no error)=w247) -> (queue out=w246:refnum<queue>, error out=w245:errorcluster)  [unwired: 1 in, 1 out]
            n95 = Enqueue Element(queue=w246, element=calib."results", error in (no error)=w245) -> (error out=w243:errorcluster)  [unwired: 1 in, 2 out]
          }
        }
      }
      frame "error" {
      }
      frame "histogram" {
        n96 = stacked-sequence {
          seq-local: [w256 _ _ _ _ _ _] -> [_ w299 _ w312 w316 w324 _]
          seq-local: [_ w298 _ _ _ _ _] -> [_ _ w305 _ _ _ _]
          seq-local: [_ _ w303 _ _ _ _] -> [_ _ _ w311 w315 w323 _]
          tunnel: "Sensor & Phase" -> [w255 _ _ _ _ _ _]
          tunnel: w254 -> [_ _ _ _ _ _ w333]
          tunnel: [_ _ _ _ _ _ w332] -> w251
          tunnel: w253 -> [_ _ _ _ _ _ w331]
          frame #0 {
            n97 = local read "Ring"() -> (w257:u16)
            n98 = case shown="\"Analog (Decreasing Values)\", Default" w255 {
              tunnel: [w258 w268 w278 w288] -> w256
              tunnel: w257 -> [w259 w269 w279 w289]
              frame "Analog (Decreasing Values)", Default {
                n99 = local read "Analog Discesa"() -> (w260:dbl[][])
                n100 = Not Equal To 0?(x=w259) -> (x != 0?=w261:bool)
                n101 = case shown="False" w261 {
                  tunnel: w260 -> [w264 w267]
                  tunnel: [w262 w266] -> w258
                  frame False {
                    n102 = Array Subset(array=w264, length (row)=100 ("length")) -> (w262:dbl[][])  [unwired: 3 in]
                  }
                  frame True {
                    n103 = Array Subset(array=w267, index (row)=100 ("length")) -> (w266:dbl[][])  [unwired: 3 in]
                  }
                }
              }
              frame "Digital (Decreasing Values)" {
                n104 = local read "Digital Discesa"() -> (w270:dbl[][])
                n105 = Not Equal To 0?(x=w269) -> (x != 0?=w271:bool)
                n106 = case shown="False" w271 {
                  tunnel: w270 -> [w274 w277]
                  tunnel: [w272 w276] -> w268
                  frame False {
                    n107 = Array Subset(array=w274, length (row)=100 ("length")) -> (w272:dbl[][])  [unwired: 3 in]
                  }
                  frame True {
                    n108 = Array Subset(array=w277, index (row)=100 ("length")) -> (w276:dbl[][])  [unwired: 3 in]
                  }
                }
              }
              frame "Digital (Increasing Values)" {
                n109 = local read "Digital Salita"() -> (w280:dbl[][])
                n110 = Not Equal To 0?(x=w279) -> (x != 0?=w281:bool)
                n111 = case shown="False" w281 {
                  tunnel: w280 -> [w284 w287]
                  tunnel: [w282 w286] -> w278
                  frame False {
                    n112 = Array Subset(array=w284, length (row)=100 ("length")) -> (w282:dbl[][])  [unwired: 3 in]
                  }
                  frame True {
                    n113 = Array Subset(array=w287, index (row)=100 ("length")) -> (w286:dbl[][])  [unwired: 3 in]
                  }
                }
              }
              frame "Analog (Increasing Values)" {
                n114 = local read "Analog Salita"() -> (w290:dbl[][])
                n115 = Not Equal To 0?(x=w289) -> (x != 0?=w291:bool)
                n116 = case shown="False" w291 {
                  tunnel: w290 -> [w294 w297]
                  tunnel: [w292 w296] -> w288
                  frame False {
                    n117 = Array Subset(array=w294, length (row)=100 ("length")) -> (w292:dbl[][])  [unwired: 3 in]
                  }
                  frame True {
                    n118 = Array Subset(array=w297, index (row)=100 ("length")) -> (w296:dbl[][])  [unwired: 3 in]
                  }
                }
              }
            }
          }
          frame #1 {
            n119 = local read "Input Sequence"() -> (w301:dbl[])
            n120 = Array Size(array=w301) -> (size(s)=w300:i32)
            n121 = call "histogram.vi"("Steps"=w300, "intervals"="Histogram intervals", "Data"=w299) -> ("Array"=w298:cluster{"X Values":dbl[], dbl[]}[][])
          }
          frame #2 {
            n122 = Decimal String To Number(string="index") -> (number=w303:i32)  [unwired: 2 in, 1 out]
            n123 = Index Array(array=w305, index (row)=w303) -> (element=→"Histogram":cluster{"X Values":dbl[], dbl[]}[])  [unwired: 1 in]
          }
          frame #3 {
            n124 = Index Array(array=w312, index (col)=w311) -> (element=w307:dbl[])  [unwired: 1 in]
            n125 = call <vilib>:"Std Deviation and Variance.vi"("X"=w307, "Weighting (Sample)"=enum16{"Sample", "Population"}."Sample") -> ("mean"=→"Mean":dbl, "standard deviation"=→"Standard Deviation":dbl)  [unwired: 1 out]
          }
          frame #4 {
            w318 = 10.0 ("Width per Box Plot")
            n126 = Index Array(array=w316, index (col)=w315) -> (element=w319:dbl[])  [unwired: 1 in]
            n127 = Bundle(w319) -> (w313:cluster{dbl[]})  [unwired: 1 in]
            n128 = Build Array(w313) -> (w314:cluster{dbl[]}[])
            n129 = call "create_plot.vi"("Width per Box Plot"=w318, "Raw Box Plot Data"=w314) -> ("Number of Plots"=w321:i32, "Box Plots"=→"Box Plot":cluster{dbl[], dbl[]}[])  [unwired: 8 in]
            n130 = control-ref of="Box Plot"() -> (w322:refnum<vi>)
            n131 = call "format_plot.vi"("Box Plot Width"=w318, "Line Color"=u32 0, "Number of Plots"=w321, "XY Graph"=w322) -> ()  [unwired: 7 in, 1 out]
          }
          frame #5 {
            n132 = Index Array(array=w324, index (col)=w323) -> (element=w325:dbl[])  [unwired: 1 in]
            n133 = call "mediano.vi"("data"=w325) -> ("Q3"=w328:dbl, "median"=w329:dbl, "Q1"=w330:dbl)  [unwired: 8 in]
            "Median" <- w329
            "Q3" <- w328
            "Q1" <- w330
            n134 = call "whisky.vi"("Median"=w329, "Lower Quartile (LQ)"=w330, "Upper Quartile (UQ)"=w328) -> ("L1"=→"L1":dbl, "U1"=→"U1":dbl)  [unwired: 1 in, 2 out]
          }
          frame #6 {
            n135 = Enqueue Element(queue=w331, element=calib."simulate", error in (no error)=w333) -> (error out=w332:errorcluster)  [unwired: 1 in, 2 out]
          }
        }
      }
      frame "results" {
        n136 = stacked-sequence {
          tunnel: w337 -> [_ _ w366]
          tunnel: w336 -> [_ _ w365]
          tunnel: [_ _ w364] -> w335
          frame #0 {
            n137 = local read "analog_salita_1"() -> (w350:dbl[][])
            n138 = local read "Analog Salita"() -> (w342:dbl[][])
            n139 = local read "analog_salita_2"() -> (w345:dbl[][])
            n140 = call "mead_and_deviation.vi"("insieme"=w350) -> ("Media"=w346:dbl[])  [unwired: 3 in, 1 out]
            n141 = call "mead_and_deviation.vi"("insieme"=w342) -> ("Dev"=→"Standard Deviations FS-1012 (mV)":dbl[], "Media"=→"Expected Values FS-1012 (mV)":dbl[])  [unwired: 3 in]
            n142 = local read "Digital Salita"() -> (w349:dbl[][])
            n143 = call "mead_and_deviation.vi"("insieme"=w345) -> ("Media"=w343:dbl[])  [unwired: 3 in, 1 out]
            n144 = call "mead_and_deviation.vi"("insieme"=w349) -> ("Dev"=→"Standard Deviations FS-2012 (mL/min)":dbl[], "Media"=w338:dbl[])  [unwired: 3 in]
            "Expected Values FS-2012 (mL/min)" <- w338
            n145 = Bundle("Media"=w338, "Media"=w346) -> (w348:cluster{"Media":dbl[], "Media":dbl[]})  [unwired: 1 in]
            n146 = Bundle("Media"=w338, "Media"=w343) -> (w344:cluster{"Media":dbl[], "Media":dbl[]})  [unwired: 1 in]
            n147 = Build Array(w348, w344) -> (→"FS-1012 Ascending & Descending Curves":cluster{"Media":dbl[], "Media":dbl[]}[])
          }
          frame #1 {
            n148 = local read "analog_discesa_1"() -> (w363:dbl[][])
            n149 = local read "Analog Discesa"() -> (w355:dbl[][])
            n150 = local read "analog_discesa_2"() -> (w358:dbl[][])
            n151 = local read "Digital Discesa"() -> (w362:dbl[][])
            n152 = call "mead_and_deviation.vi"("insieme"=w363) -> ("Media"=w359:dbl[])  [unwired: 3 in, 1 out]
            n153 = call "mead_and_deviation.vi"("insieme"=w355) -> ("Dev"=→"stdad":dbl[], "Media"=→"exad":dbl[])  [unwired: 3 in]
            n154 = call "mead_and_deviation.vi"("insieme"=w358) -> ("Media"=w357:dbl[])  [unwired: 3 in, 1 out]
            n155 = call "mead_and_deviation.vi"("insieme"=w362) -> ("Dev"=→"stddd":dbl[], "Media"=w351:dbl[])  [unwired: 3 in]
            "exdd" <- w351
            n156 = Bundle("Media"=w351, "Media"=w359) -> (w360:cluster{"Media":dbl[], "Media":dbl[]})  [unwired: 1 in]
            n157 = Bundle("Media"=w351, "Media"=w357) -> (w356:cluster{"Media":dbl[], "Media":dbl[]})  [unwired: 1 in]
            n158 = Build Array(w360, w356) -> (→"FS-2012 Ascending & Descending Curves":cluster{"Media":dbl[], "Media":dbl[]}[])
          }
          frame #2 {
            n159 = Enqueue Element(queue=w366, element=calib."results2", error in (no error)=w365) -> (queue out=w367:refnum<queue>, error out=w370:errorcluster)  [unwired: 1 in, 1 out]
            n160 = Enqueue Element(queue=w367, element=calib."comparison", error in (no error)=w370) -> (error out=w364:errorcluster)  [unwired: 1 in, 2 out]
          }
        }
      }
      frame "results2" {
        n161 = local read "Digital Discesa"() -> (w376:dbl[][])
        n162 = local read "Digital Salita"() -> (w377:dbl[][])
        n163 = Enqueue Element(queue=w374, element=calib."result3", error in (no error)=w373) -> (error out=w371:errorcluster)  [unwired: 1 in, 2 out]
        n164 = Build Array (concatenate)(w376, w377) -> (→"total_flow":dbl[][])
      }
      frame "result3" {
        n165 = stacked-sequence {
          seq-local: [w383 _ _ _] -> [_ w394 _ _]
          seq-local: [w384 _ _ _] -> [_ w393 _ _]
          seq-local: [w382 _ _ _] -> [_ _ w404 _]
          seq-local: [w381 _ _ _] -> [_ _ w403 _]
          tunnel: w380 -> [_ _ _ w408]
          tunnel: w379 -> [_ _ _ w406]
          tunnel: [_ _ _ w405] -> w378
          frame #0 {
            n166 = local read "Digital Discesa"() -> (w381:dbl[][])
            n167 = local read "Digital Salita"() -> (w382:dbl[][])
            n168 = local read "Analog Discesa"() -> (w384:dbl[][])
            n169 = local read "Analog Salita"() -> (w383:dbl[][])
          }
          frame #1 {
            n170 = call "uncertainty_datasets.vi"("Discesa"=w393, "Salita"=w394) -> ("uncertainty ascending phase (point-by-point)"=→"uncaa":dbl[], "uncertainty descending phase (point-by-point)"=→"uncad":dbl[], "Maximum uncertainty Descending Phase"=w388:dbl, "Maximum uncertainty Ascending Phase"=w389:dbl)  [unwired: 2 in]
            n171 = Multiply(x=w389, y=2.0) -> (x*y=→"Max Uncertainty\n (Ascending) [mV]":dbl)
            n172 = Multiply(x=w388, y=2.0) -> (x*y=→"Max Uncertainty\n (Descending) [mV]":dbl)
          }
          frame #2 {
            n173 = call "uncertainty_datasets.vi"("Discesa"=w403, "Salita"=w404) -> ("uncertainty ascending phase (point-by-point)"=→"uncda":dbl[], "uncertainty descending phase (point-by-point)"=→"uncdd":dbl[], "Maximum uncertainty Descending Phase"=w398:dbl, "Maximum uncertainty Ascending Phase"=w399:dbl)  [unwired: 2 in]
            n174 = Multiply(x=w399, y=2.0) -> (x*y=→"Max Uncertainty\n (Ascending) [mL/min]\n\n2":dbl)
            n175 = Multiply(x=w398, y=2.0) -> (x*y=→"Max Uncertainty\n (Descending) [mL/min]\n\n2":dbl)
          }
          frame #3 {
            n176 = Enqueue Element(queue=w408, element=calib."results4", error in (no error)=w406) -> (error out=w405:errorcluster)  [unwired: 1 in, 2 out]
          }
        }
      }
      frame "results4" {
        n177 = stacked-sequence {
          tunnel: w411 -> [_ _ w430]
          tunnel: w410 -> [_ _ w428]
          tunnel: [_ _ w425] -> w409
          frame #0 {
            n178 = local read "Max Uncertainty\n (Descending) [mV]"() -> (w413:dbl)
            n179 = local read "Max Uncertainty\n (Ascending) [mV]"() -> (w416:dbl)
            n180 = Square(x=w416) -> (x^2=w415:dbl)
            n181 = Square(x=w413) -> (x^2=w414:dbl)
            n182 = Add(x=w415, y=w414) -> (x+y=w417:dbl)
            n183 = Square Root(x=w417) -> (sqrt(x)=→"Max Combined \nUncertainty (RSS) [mV]":dbl)
          }
          frame #1 {
            n184 = local read "Max Uncertainty\n (Descending) [mL/min]\n\n2"() -> (w422:dbl)
            n185 = local read "Max Uncertainty\n (Ascending) [mL/min]\n\n2"() -> (w421:dbl)
            n186 = Square(x=w421) -> (x^2=w419:dbl)
            n187 = Square(x=w422) -> (x^2=w418:dbl)
            n188 = Add(x=w419, y=w418) -> (x+y=w420:dbl)
            n189 = Square Root(x=w420) -> (sqrt(x)=→"Max Combined \nUncertainty (RSS) [mL/min]\n\n2":dbl)
          }
          frame #2 {
            n190 = Enqueue Element(queue=w430, element=calib."curves", error in (no error)=w428) -> (queue out=w427:refnum<queue>, error out=w426:errorcluster)  [unwired: 1 in, 1 out]
            n191 = Enqueue Element(queue=w427, element=calib."comparison", error in (no error)=w426) -> (error out=w425:errorcluster)  [unwired: 1 in, 2 out]
          }
        }
      }
      frame "comparison" {
      }
      frame "curves" {
        n192 = stacked-sequence {
          seq-local: [w436 _ _ _ _] -> [_ w443 _ _ _]
          seq-local: [w435 _ _ _ _] -> [_ _ w451 _ _]
          seq-local: [w434 _ _ _ _] -> [_ w442 _ _ _]
          seq-local: [w433 _ _ _ _] -> [_ _ w450 _ _]
          seq-local: [_ w439 _ _ _] -> [_ _ w445 _ _]
          seq-local: [_ _ w444 _ _] -> [_ _ _ w457 _]
          tunnel: w432 -> [_ _ _ w456 _]
          tunnel: w431 -> [_ _ _ w454 _]
          tunnel: [_ _ _ w453 _] -> _
          frame #0 {
            n193 = local read "Analog Discesa"() -> (w435:dbl[][])
            n194 = local read "Analog Salita"() -> (w436:dbl[][])
            n195 = local read "Digital Discesa"() -> (w433:dbl[][])
            n196 = local read "Digital Salita"() -> (w434:dbl[][])
          }
          frame #1 {
            # "Ascending Table"
            n197 = call "mead_and_deviation.vi"("insieme"=w443) -> ("Media"=w437:dbl[])  [unwired: 3 in, 1 out]
            n198 = call "mead_and_deviation.vi"("insieme"=w442) -> ("Media"=w438:dbl[])  [unwired: 3 in, 1 out]
            n199 = Build Array "Build Array"(w437, w438) -> (w441:dbl[][])
            n200 = Bundle("Media"=w438, "Media"=w437) -> (w439:cluster{"Media":dbl[], "Media":dbl[]})  [unwired: 1 in]
            n201 = Transpose 2D Array(2D array=w441) -> (transposed array=→"Ascending Table":dbl[][])
          }
          frame #2 {
            # "Descending Table"
            n202 = call "mead_and_deviation.vi"("insieme"=w451) -> ("Media"=w447:dbl[])  [unwired: 3 in, 1 out]
            n203 = call "mead_and_deviation.vi"("insieme"=w450) -> ("Media"=w448:dbl[])  [unwired: 3 in, 1 out]
            n204 = Build Array(w447, w448) -> (w452:dbl[][])
            n205 = Bundle("Media"=w448, "Media"=w447) -> (w446:cluster{"Media":dbl[], "Media":dbl[]})  [unwired: 1 in]
            n206 = Build Array(w445, w446) -> (w444:cluster{"Media":dbl[], "Media":dbl[]}[])
            n207 = Transpose 2D Array(2D array=w452) -> (transposed array=→"Descending Table":dbl[][])
          }
          frame #3 {
            n208 = Enqueue Element(queue=w456, element=calib."fitting", error in (no error)=w454) -> (error out=w453:errorcluster)  [unwired: 1 in, 2 out]
            "COMPARISON" <- w457
          }
          frame #4 {
          }
        }
      }
      frame "linear regression" {
        n209 = stacked-sequence {
          seq-local: [w462 _ _ _ _ _ _ _ _] -> [_ w472 _ _ _ _ _ _ _]
          seq-local: [w463 _ _ _ _ _ _ _ _] -> [_ w471 _ _ _ _ _ _ _]
          seq-local: [_ w470 _ _ _ _ _ _ _] -> [_ _ w474 w491 _ _ w520 _ _]
          seq-local: [_ w469 _ _ _ _ _ _ _] -> [_ _ w475 _ _ _ w519 _ _]
          seq-local: [_ _ w478 _ _ _ _ _ _] -> [_ _ _ w494 _ _ w518 _ _]
          seq-local: [_ _ w477 _ _ _ _ _ _] -> [_ _ _ _ w495 _ _ _ _]
          seq-local: [_ _ w476 _ _ _ _ _ _] -> [_ _ _ _ w496 _ _ _ _]
          seq-local: [_ _ _ _ w500 _ _ _ _] -> [_ _ _ _ _ w503 _ _ _]
          seq-local: [_ _ _ _ w499 _ _ _ _] -> [_ _ _ _ _ w502 _ _ _]
          seq-local: [_ _ _ _ _ _ w521 _ _] -> [_ _ _ _ _ _ _ w525 _]
          tunnel: "Tab Control 9" -> [w464 _ w473 _ _ w501 _ w524 _]
          tunnel: w460 -> [_ _ _ _ _ _ _ _ w530]
          tunnel: w459 -> [_ _ _ _ _ _ _ _ w529]
          tunnel: [_ _ _ _ _ _ _ _ w531] -> w458
          frame #0 {
            n210 = case shown="\"Ascending (Voltage vs. Flow)\", Default" w464 {
              tunnel: [w466 w468] -> w462
              tunnel: [w465 w467] -> w463
              frame "Ascending (Voltage vs. Flow)", Default {
                n211 = local read "Analog Salita"() -> (w466:dbl[][])
                n212 = local read "Digital Salita"() -> (w465:dbl[][])
              }
              frame "Descending (Voltage vs. Flow)" {
                n213 = local read "Analog Discesa"() -> (w468:dbl[][])
                n214 = local read "Digital Discesa"() -> (w467:dbl[][])
              }
            }
          }
          frame #1 {
            n215 = call "mead_and_deviation.vi"("insieme"=w472) -> ("Media"=w470:dbl[])  [unwired: 3 in, 1 out]
            n216 = call "mead_and_deviation.vi"("insieme"=w471) -> ("Media"=w469:dbl[])  [unwired: 3 in, 1 out]
          }
          frame #2 {
            n217 = case shown="\"Ascending (Voltage vs. Flow)\", Default" w473 {
              tunnel: [w483 w489] -> w478
              tunnel: [w482 w488] -> w477
              tunnel: [w481 w487] -> w476
              tunnel: w475 -> [w480 w486]
              tunnel: w474 -> [w479 w485]
              frame "Ascending (Voltage vs. Flow)", Default {
                w484 = T15 0 items=["Least Square", "Least Absolute Residual", "Bisquare"] ("method")
                n218 = call <vilib>:"Linear Fit.vi"("Y"=w479, "X"=w480, "method"=w484) -> ("Best Linear Fit"=w483:dbl[], "slope"=w482:dbl, "intercept"=w481:dbl)  [unwired: 8 in, 2 out]
                "Best Linear Fit A" <- w483
              }
              frame "Descending (Voltage vs. Flow)" {
                w490 = T15 0 items=["Least Square", "Least Absolute Residual", "Bisquare"] ("method")
                n219 = call <vilib>:"Linear Fit.vi"("Y"=w485, "X"=w486, "method"=w490) -> ("Best Linear Fit"=w489:dbl[], "slope"=w488:dbl, "intercept"=w487:dbl)  [unwired: 8 in, 2 out]
                "Best Linear Fit D" <- w489
              }
            }
          }
          frame #3 {
            n220 = call <vilib>:"Goodness of Fit.vi"("Best Fit"=w494, "Y"=w491) -> ("RMSE"=→"RMSE 2":dbl, "R-square"=→"R_sqr":dbl)  [unwired: 6 in, 2 out]
          }
          frame #4 {
            n221 = Number To Fractional String(number=w495, precision (6)=i16 3) -> (F-format string=w500:string)  [unwired: 2 in]
            n222 = Number To Fractional String(number=w496, precision (6)=i16 1) -> (F-format string=w499:string)  [unwired: 2 in]
            "b" <- w496
            "m" <- w495
          }
          frame #5 {
            n223 = case shown="\"Descending (Voltage vs. Flow)\", Default" w501 {
              tunnel: w503 -> [w506 w512]
              tunnel: w502 -> [w505 w511]
              frame "Descending (Voltage vs. Flow)", Default {
                n224 = Concatenate Strings(" = " ("string"), w506, " *F + " ("string"), w505) -> (w510:string)
                n225 = Concatenate Strings("V" ("symb"), w510) -> (→"eqD":string)
              }
              frame "Ascending (Voltage vs. Flow)" {
                n226 = Concatenate Strings(" = " ("string"), w512, " *F + " ("string"), w511) -> (w517:string)
                n227 = Concatenate Strings("V" ("symb"), w517) -> (→"eqA":string)
              }
            }
          }
          frame #6 {
            n228 = Bundle("Media"=w519, "Media"=w520) -> (w522:cluster{"Media":dbl[], "Media":dbl[]})  [unwired: 1 in]
            n229 = Bundle("Media"=w519, "Best Linear Fit"=w518) -> (w523:cluster{"Media":dbl[], "Best Linear Fit":dbl[]})  [unwired: 1 in]
            n230 = Build Array(w522, w523) -> (w521:T16)
            "Best Linear Fit D2" <- w518
          }
          frame #7 {
            n231 = case shown="\"Ascending (Voltage vs. Flow)\", Default" w524 {
              tunnel: w525 -> [w526 w527]
              frame "Ascending (Voltage vs. Flow)", Default {
                "A" <- w526
              }
              frame "Descending (Voltage vs. Flow)" {
                "D" <- w527
              }
            }
          }
          frame #8 {
            n232 = Enqueue Element(queue=w530, element=calib."combined uncertainty", error in (no error)=w529) -> (error out=w531:errorcluster)  [unwired: 1 in, 2 out]
          }
        }
      }
      frame "linearization" {
        n233 = local read "Tab Control 9"() -> (w535:T9)
        n234 = stacked-sequence {
          seq-local: [w540 _ _ _ _] -> [_ w559 _ _ _]
          seq-local: [w539 _ _ _ _] -> [_ w560 _ _ _]
          seq-local: [w538 _ _ _ _] -> [_ w565 _ _ _]
          seq-local: [w537 _ _ _ _] -> [_ _ w569 _ _]
          seq-local: [w536 _ _ _ _] -> [_ w562 _ _ _]
          seq-local: [_ w563 _ _ _] -> [_ _ w568 w586 _]
          seq-local: [_ w558 _ _ _] -> [_ _ w566 w587 _]
          tunnel: w535 -> [w541 _ w567 w582 _]
          tunnel: w534 -> [_ _ _ _ w608]
          tunnel: w533 -> [_ _ _ _ w607]
          tunnel: [_ _ _ _ w605] -> w532
          frame #0 {
            n235 = case shown="\"Descending (Flow in vs. Flow out)\"" w541 {
              tunnel: [w548 w556] -> w540
              tunnel: [w547 w555] -> w539
              tunnel: [w545 w553] -> w538
              tunnel: [w543 w551] -> w537
              tunnel: [w542 w550] -> w536
              frame "Descending (Flow in vs. Flow out)" {
                n236 = local read "Digital Discesa"() -> (w544:dbl[][])
                n237 = local read "Analog Discesa"() -> (w546:dbl[][])
                n238 = local read "eqD"() -> (w549:string)
                n239 = call "mead_and_deviation.vi"("insieme"=w544) -> ("Media"=w543:dbl[])  [unwired: 3 in, 1 out]
                n240 = call "scan_equation.vi"("Equation"=w549) -> ("Intercept"=w547:dbl, "Angular Coefficient"=w548:dbl)  [unwired: 3 in]
                n241 = call "mead_and_deviation.vi"("insieme"=w546) -> ("Media"=w545:dbl[])  [unwired: 3 in, 1 out]
                n242 = local read "Best Linear Fit D2"() -> (w542:dbl[])
              }
              frame "Ascending (Flow in vs. Flow Out)", Default {
                n243 = local read "Digital Salita"() -> (w552:dbl[][])
                n244 = local read "Analog Salita"() -> (w554:dbl[][])
                n245 = local read "eqA"() -> (w557:string)
                n246 = call "mead_and_deviation.vi"("insieme"=w552) -> ("Media"=w551:dbl[])  [unwired: 3 in, 1 out]
                n247 = call "scan_equation.vi"("Equation"=w557) -> ("Intercept"=w555:dbl, "Angular Coefficient"=w556:dbl)  [unwired: 3 in]
                n248 = call "mead_and_deviation.vi"("insieme"=w554) -> ("Media"=w553:dbl[])  [unwired: 3 in, 1 out]
                n249 = local read "Best Linear Fit A"() -> (w550:dbl[])
              }
            }
          }
          frame #1 {
            n250 = Subtract(x=w565, y=w560) -> (x-y=w564:dbl[])
            n251 = Divide(x=w564, y=w559) -> (x/y=w563:dbl[])
            n252 = Subtract(x=w562, y=w560) -> (x-y=w561:dbl[])
            n253 = Divide(x=w561, y=w559) -> (x/y=w558:dbl[])
          }
          frame #2 {
            n254 = case shown="\"Ascending (Flow in vs. Flow Out)\", Default" w567 {
              tunnel: w569 -> [w573 w579]
              tunnel: w568 -> [w575 w581]
              tunnel: w566 -> [w574 w580]
              frame "Ascending (Flow in vs. Flow Out)", Default {
                n255 = Bundle("Media"=w573, w575) -> (w572:cluster{"Media":dbl[], dbl[]})  [unwired: 1 in]
                n256 = Bundle("Media"=w573, w574) -> (w571:cluster{"Media":dbl[], dbl[]})  [unwired: 1 in]
                n257 = Build Array(w572, w571) -> (→"A 2":cluster{"Media":dbl[], dbl[]}[])
                "Estimate Ascending" <- w575
              }
              frame "Descending (Flow in vs. Flow out)" {
                n258 = Bundle("Media"=w579, w581) -> (w578:cluster{"Media":dbl[], dbl[]})  [unwired: 1 in]
                n259 = Bundle("Media"=w579, w580) -> (w577:cluster{"Media":dbl[], dbl[]})  [unwired: 1 in]
                n260 = Build Array(w578, w577) -> (→"D 2":cluster{"Media":dbl[], dbl[]}[])
                "Estimate Descending" <- w581
              }
            }
          }
          frame #3 {
            # "table of linearization biases"
            n261 = case shown="\"Descending (Flow in vs. Flow out)\"" w582 {
              tunnel: [w596 w604] -> w588
              tunnel: w587 -> [w594 w602]
              tunnel: w586 -> [w593 w601]
              tunnel: [w592 w600] -> w583
              frame "Ascending (Flow in vs. Flow Out)", Default {
                n262 = Subtract(x=w594, y=w593) -> (x-y=w589:dbl[])
                n263 = Array Max & Min(array=w593) -> ()  [unwired: 4 out]
                n264 = Build Array(w594, w593, w589) -> (w595:dbl[][])
                n265 = Array Max & Min(array=w589) -> (max value=w590:dbl)  [unwired: 3 out]
                n266 = Transpose 2D Array(2D array=w595) -> (transposed array=w596:dbl[][])
                "asc_table" <- w596
                n267 = Divide(x=w590, y=10000.0) -> (x/y=w592:dbl)
              }
              frame "Descending (Flow in vs. Flow out)" {
                n268 = Subtract(x=w602, y=w601) -> (x-y=w598:dbl[])
                n269 = Array Max & Min(array=w601) -> ()  [unwired: 4 out]
                n270 = Build Array(w602, w601, w598) -> (w603:dbl[][])
                n271 = Array Max & Min(array=w598) -> (max value=w597:dbl)  [unwired: 3 out]
                n272 = Transpose 2D Array(2D array=w603) -> (transposed array=w604:dbl[][])
                "disc_table 2" <- w604
                n273 = Divide(x=w597, y=10000.0) -> (x/y=w600:dbl)
              }
            }
            "Ascending Table 2" <- w588
            n274 = Multiply(x=w583, y=100.0) -> (x*y=→"nonlinearity":dbl)
          }
          frame #4 {
            n275 = Enqueue Element(queue=w608, element=calib."calibration curve", error in (no error)=w607) -> (error out=w605:errorcluster)  [unwired: 1 in, 2 out]
          }
        }
      }
      frame "calibration curve" {
        n276 = stacked-sequence {
          seq-local: [w617 _ _ _ _ _ _ _ _ _ _] -> [_ w629 _ _ _ _ _ w665 _ _ _]
          seq-local: [w613 _ _ _ _ _ _ _ _ _ _] -> [_ w623 _ _ _ _ _ _ _ _ _]
          seq-local: [w614 _ _ _ _ _ _ _ _ _ _] -> [_ w625 _ _ _ _ _ _ _ _ _]
          seq-local: [_ w627 _ _ _ _ _ _ _ _ _] -> [_ _ _ _ _ _ _ w672 w673 _ _]
          seq-local: [_ w622 _ _ _ _ _ _ _ _ _] -> [_ _ _ _ _ _ _ w669 w681 _ _]
          seq-local: [w612 _ _ _ _ _ _ _ _ _ _] -> [_ _ _ _ _ _ _ _ _ _ _]
          tunnel: w611 -> [_ _ _ _ _ _ _ _ _ _ w737]
          tunnel: w610 -> [_ _ _ _ _ _ _ _ _ _ w736]
          tunnel: [_ _ _ _ _ _ _ _ _ _ w735] -> w609
          frame #0 {
            w618 = T15 0 items=["Least Square", "Least Absolute Residual", "Bisquare"] ("method")
            # "Compute Average values curve.\nThen estimate the linear regressor from the average values."
            n277 = local read "Analog Discesa"() -> (w620:dbl[][])
            n278 = local read "Analog Salita"() -> (w621:dbl[][])
            n279 = local read "total_flow"() -> (w619:dbl[][])
            n280 = Build Array (concatenate)(w621, w620) -> (w612:dbl[][])
            n281 = call "mead_and_deviation.vi"("insieme"=w612) -> ("Media"=w616:dbl[])  [unwired: 3 in, 1 out]
            "Media" <- w616
            n282 = call "mead_and_deviation.vi"("insieme"=w619) -> ("Media"=w615:dbl[])  [unwired: 3 in, 1 out]
            "Media 2" <- w615
            n283 = call <vilib>:"Linear Fit.vi"("Y"=w616, "X"=w615, "method"=w618) -> ("Best Linear Fit"=w617:dbl[], "slope"=w613:dbl, "intercept"=w614:dbl)  [unwired: 8 in, 2 out]
            "b avg" <- w614
            "m avg" <- w613
          }
          frame #1 {
            n284 = local read "Media"() -> (w626:dbl[])
            n285 = Subtract(x=w626, y=w625) -> (x-y=w624:dbl[])
            n286 = Divide(x=w624, y=w623) -> (x/y=w622:dbl[])
            n287 = Subtract(x=w629, y=w625) -> (x-y=w628:dbl[])
            n288 = Divide(x=w628, y=w623) -> (x/y=w627:dbl[])
          }
          frame #2 {
          }
          frame #3 {
            n289 = local read "disc_table 2"() -> (w631:dbl[][])
            n290 = local read "asc_table"() -> (w632:dbl[][])
            n291 = Index Array(array=w632, index (col)=1 ("disabled index (col)")) -> (element=w636:dbl[])  [unwired: 1 in]
            n292 = Index Array(array=w631, index (col)=1 ("disabled index (col)")) -> (element=w635:dbl[])  [unwired: 1 in]
            n293 = Subtract(x=w636, y=w635) -> (x-y=w634:dbl[])
            "difference" <- w634
            n294 = Absolute Value(x=w634) -> (abs(x)=w633:dbl[])
            "abs(x)" <- w633
            n295 = Array Max & Min(array=w633) -> (max value=→"Max Deviation":dbl)  [unwired: 3 out]
          }
          frame #4 {
            n296 = local read "Max Uncertainty\n (Descending) [mV]"() -> (w645:dbl)
            n297 = local read "Max Uncertainty\n (Ascending) [mV]"() -> (w646:dbl)
            n298 = local read "m avg"() -> (w639:dbl)
            n299 = Square(x=w646) -> (x^2=w644:dbl)
            n300 = Square(x=w645) -> (x^2=w643:dbl)
            n301 = Add(x=w644, y=w643) -> (x+y=w642:dbl)
            n302 = Square Root(x=w642) -> (sqrt(x)=w641:dbl)
            n303 = Divide(x=w641, y=w639) -> (x/y=→"Max Uncertainty":dbl)
          }
          frame #5 {
            n304 = local read "Max Deviation"() -> (w649:dbl)
            n305 = Divide(x=w649, y=10000.0) -> (x/y=w650:dbl)
            n306 = Multiply(x=w650, y=100.0) -> (x*y=→"Hysteresis %FSO":dbl)
          }
          frame #6 {
            n307 = local read "Max Uncertainty"() -> (w654:dbl)
            n308 = local read "Max Deviation"() -> (w653:dbl)
            n309 = Square(x=w654) -> (x^2=w656:dbl)
            n310 = Square(x=w653) -> (x^2=w657:dbl)
            n311 = Add(x=w656, y=w657) -> (x+y=w655:dbl)
            n312 = Square Root(x=w655) -> (sqrt(x)=→"x/y":dbl)
          }
          frame #7 {
            n313 = Subtract(x=w669, y=w672) -> (x-y=w671:dbl[])
            n314 = Absolute Value(x=w671) -> (abs(x)=w661:dbl[])
            n315 = Square(x=w661) -> (x^2=w660:dbl[])
            n316 = Array Max & Min(array=w661) -> (max value=w670:dbl)  [unwired: 3 out]
            "max value" <- w670
            n317 = local read "Media"() -> (w664:dbl[])
            n318 = Add Array Elements(numeric array=w660) -> (sum=→"sum of squared errors":dbl)
            n319 = Divide(x=w670, y=10000.0) -> (x/y=w668:dbl)
            n320 = call <vilib>:"Goodness of Fit.vi"("Best Fit"=w665, "Y"=w664) -> ("RMSE"=→"R-square avg":dbl, "R-square"=→"RMSE_avg":dbl)  [unwired: 6 in, 2 out]
            n321 = Multiply(x=w668, y=100.0) -> (x*y=→"Nonlinearity %FSO":dbl)
          }
          frame #8 {
            n322 = local read "total_flow"() -> (w692:dbl[][])
            n323 = call "mead_and_deviation.vi"("insieme"=w692) -> ("Media"=w674:dbl[])  [unwired: 3 in, 1 out]
            n324 = local read "Estimate Descending"() -> (w679:dbl[])
            n325 = local read "Estimate Ascending"() -> (w680:dbl[])
            n326 = local read "x/y"() -> (w688:dbl)
            n327 = Add(x=w681, y=w688) -> (x+y=w687:dbl[])
            n328 = Subtract(x=w681, y=w688) -> (x-y=w686:dbl[])
            n329 = Bundle(w673, "Media"=w674) -> (w691:cluster{dbl[], "Media":dbl[]})  [unwired: 1 in]
            n330 = Bundle(w673, w687) -> (w685:cluster{dbl[], dbl[]})  [unwired: 1 in]
            n331 = Bundle(w673, w686) -> (w684:cluster{dbl[], dbl[]})  [unwired: 1 in]
            n332 = Bundle(w673, w681) -> (w689:cluster{dbl[], dbl[]})  [unwired: 1 in]
            n333 = Bundle(w673, "Estimate Ascending"=w680) -> (w683:cluster{dbl[], "Estimate Ascending":dbl[]})  [unwired: 1 in]
            n334 = Bundle(w673, "Estimate Descending"=w679) -> (w682:cluster{dbl[], "Estimate Descending":dbl[]})  [unwired: 1 in]
            n335 = Bundle("Media"=w674, "Estimate Descending"=w679) -> (w678:T17)  [unwired: 1 in]
            n336 = Bundle("Media"=w674, "Estimate Ascending"=w680) -> (w677:T18)  [unwired: 1 in]
            n337 = Bundle("Media"=w674, w673) -> (w676:cluster{"Media":dbl[], dbl[]})  [unwired: 1 in]
            n338 = Build Array(w691, w685, w684, w689, w683, w682) -> (→"Calibration Curve":cluster{dbl[], "Estimate Descending":dbl[]}[])
            n339 = Build Array(w678, w677, w676) -> (→"Hysteresis Graph":T19)
            "Array" <- w673
          }
          frame #9 {
            n340 = case shown="\"Item 0\", Default" "Plot" {
              frame "Item 0", Default {
                n341 = stacked-sequence {
                  frame #0 {
                    n342 = property on="Calibration Curve" class="XYGraph (strict)"("Active Plot"=u32 5) -> (error out=w695:errorcluster)  [unwired: 2 in, 1 out]
                    n343 = property on="Calibration Curve" class="XYGraph (strict)"("Active Plot"=u32 4) -> (error out=w698:errorcluster)  [unwired: 2 in, 1 out]
                    n344 = property on="Calibration Curve" class="XYGraph (strict)"(error in=w695, "Plot.Visible?"=TRUE ("Plot.Visible")) -> ()  [unwired: 1 in, 2 out]
                    n345 = property on="Calibration Curve" class="XYGraph (strict)"(error in=w698, "Plot.Visible?"=TRUE ("Plot.Visible")) -> ()  [unwired: 1 in, 2 out]
                  }
                  frame #1 {
                    n346 = property on="Calibration Curve" class="XYGraph (strict)"("Active Plot"=u32 3) -> (error out=w700:errorcluster)  [unwired: 2 in, 1 out]
                    n347 = property on="Calibration Curve" class="XYGraph (strict)"("Active Plot"=u32 2) -> (error out=w705:errorcluster)  [unwired: 2 in, 1 out]
                    n348 = property on="Calibration Curve" class="XYGraph (strict)"("Active Plot"=u32 2) -> (error out=w707:errorcluster)  [unwired: 2 in, 1 out]
                    n349 = property on="Calibration Curve" class="XYGraph (strict)"("Active Plot"=u32 1) -> (error out=w710:errorcluster)  [unwired: 2 in, 1 out]
                    n350 = property on="Calibration Curve" class="XYGraph (strict)"(error in=w700, "Plot.Visible?"=FALSE ("Plot.Visible")) -> ()  [unwired: 1 in, 2 out]
                    n351 = property on="Calibration Curve" class="XYGraph (strict)"(error in=w705, "Plot.Visible?"=FALSE ("Plot.Visible")) -> ()  [unwired: 1 in, 2 out]
                    n352 = property on="Calibration Curve" class="XYGraph (strict)"(error in=w707, "Plot.Visible?"=FALSE ("Plot.Visible")) -> ()  [unwired: 1 in, 2 out]
                    n353 = property on="Calibration Curve" class="XYGraph (strict)"(error in=w710, "Plot.Visible?"=FALSE ("Plot.Visible")) -> ()  [unwired: 1 in, 2 out]
                  }
                  frame #2 {
                    n354 = property on="Calibration Curve" class="XYGraph (strict)"("XScale.NameLbl.Text"="Reference Flow Rate [mL/min]" ("X Scale.Name Label.Text"), "YScale.NameLbl.Text"="DUT Flow Rate [mL/min]" ("Y Scale.Name Label.Text")) -> ()  [unwired: 2 in, 2 out]
                  }
                }
              }
              frame "Radio Selection 4" {
                n355 = stacked-sequence {
                  frame #0 {
                    n356 = property on="Calibration Curve" class="XYGraph (strict)"("Active Plot"=u32 5) -> (error out=w714:errorcluster)  [unwired: 2 in, 1 out]
                    n357 = property on="Calibration Curve" class="XYGraph (strict)"("Active Plot"=u32 4) -> (error out=w719:errorcluster)  [unwired: 2 in, 1 out]
                    n358 = property on="Calibration Curve" class="XYGraph (strict)"(error in=w714, "Plot.Visible?"=FALSE ("Plot.Visible")) -> ()  [unwired: 1 in, 2 out]
                    n359 = property on="Calibration Curve" class="XYGraph (strict)"(error in=w719, "Plot.Visible?"=FALSE ("Plot.Visible")) -> ()  [unwired: 1 in, 2 out]
                  }
                  frame #1 {
                    n360 = property on="Calibration Curve" class="XYGraph (strict)"("Active Plot"=u32 1) -> (error out=w726:errorcluster)  [unwired: 2 in, 1 out]
                    n361 = property on="Calibration Curve" class="XYGraph (strict)"("Active Plot"=u32 2) -> (error out=w725:errorcluster)  [unwired: 2 in, 1 out]
                    n362 = property on="Calibration Curve" class="XYGraph (strict)"("Active Plot"=u32 0) -> (error out=w731:errorcluster)  [unwired: 2 in, 1 out]
                    n363 = property on="Calibration Curve" class="XYGraph (strict)"("Active Plot"=u32 3) -> (error out=w720:errorcluster)  [unwired: 2 in, 1 out]
                    n364 = property on="Calibration Curve" class="XYGraph (strict)"(error in=w726, "Plot.Visible?"=TRUE ("Plot.Visible")) -> ()  [unwired: 1 in, 2 out]
                    n365 = property on="Calibration Curve" class="XYGraph (strict)"(error in=w725, "Plot.Visible?"=TRUE ("Plot.Visible")) -> ()  [unwired: 1 in, 2 out]
                    n366 = property on="Calibration Curve" class="XYGraph (strict)"(error in=w731, "Plot.Visible?"=TRUE ("Plot.Visible")) -> ()  [unwired: 1 in, 2 out]
                    n367 = property on="Calibration Curve" class="XYGraph (strict)"(error in=w720, "Plot.Visible?"=TRUE ("Plot.Visible")) -> ()  [unwired: 1 in, 2 out]
                  }
                  frame #2 {
                    n368 = property on="Calibration Curve" class="XYGraph (strict)"("XScale.NameLbl.Text"="DUT Flow Rate [mL/min]" ("Y Scale.Name Label.Text"), "YScale.NameLbl.Text"="Reference Flow Rate [mL/min]" ("X Scale.Name Label.Text")) -> ()  [unwired: 2 in, 2 out]
                  }
                }
              }
            }
          }
          frame #10 {
            n369 = Enqueue Element(queue=w737, element=calib."combined uncertainty", error in (no error)=w736) -> (error out=w735:errorcluster)  [unwired: 1 in, 2 out]
          }
        }
      }
      frame "combined uncertainty" {
        n370 = stacked-sequence {
          seq-local: [w738 _ _ _ _ _ _ _] -> [_ _ _ _ _ _ _ _]
          seq-local: [_ _ _ _ _ _ w774 _] -> [_ _ _ _ _ _ _ w789]
          seq-local: [_ w741 _ _ _ _ _ _] -> [_ _ _ _ _ _ w777 _]
          seq-local: [_ _ w750 _ _ _ _ _] -> [_ _ _ _ _ _ w776 _]
          seq-local: [_ _ _ w757 _ _ _ _] -> [_ _ _ _ _ _ w773 _]
          seq-local: [_ _ _ _ w765 _ _ _] -> [_ _ _ _ _ _ w772 _]
          seq-local: [_ _ _ _ _ w768 _ _] -> [_ _ _ _ _ _ w775 _]
          frame #0 {
            # "Average points dataset (ascending dataset V descending dataset)"
            n371 = local read "Analog Discesa"() -> (w740:dbl[][])
            n372 = local read "Analog Salita"() -> (w739:dbl[][])
            n373 = Build Array (concatenate)(w739, w740) -> (w738:dbl[][])
          }
          frame #1 {
            # "Select the max. unc. (in mL/min)"
            n374 = local read "Max Uncertainty\n (Descending) [mV]"() -> (w747:dbl)
            n375 = local read "Max Uncertainty\n (Ascending) [mV]"() -> (w748:dbl)
            n376 = local read "m avg"() -> (w742:dbl)
            n377 = Square(x=w748) -> (x^2=w746:dbl)
            n378 = Square(x=w747) -> (x^2=w745:dbl)
            n379 = Add(x=w746, y=w745) -> (x+y=w744:dbl)
            n380 = Square Root(x=w744) -> (sqrt(x)=w743:dbl)
            n381 = Divide(x=w743, y=w742) -> (x/y=w741:dbl)
          }
          frame #2 {
            # "Rectangular Distribution"
            n382 = local read "m avg"() -> (w751:dbl)
            n383 = Fract/Exp String To Number(string="DAQ Resolution") -> (number=w753:dbl)  [unwired: 3 in, 1 out]
            n384 = Square Root(x=12.0) -> (sqrt(x)=w749:dbl)
            n385 = Divide(x=w753, y=w749) -> (x/y=w752:dbl)
            "Standard Uncertainty DAQ (mV)" <- w752
            n386 = Divide(x=w752, y=w751) -> (x/y=w750:dbl)
            "Standard Uncertainty DAQ (mL/min)" <- w750
          }
          frame #3 {
            # "Accuracy of the reference sensor (FS-2012)\nis 2% of Reading (R). We choose R as the FSO."
            n387 = Multiply(x=2.0, y=10000.0) -> (x*y=w762:dbl)
            n388 = Divide(x=w762, y=100.0) -> (x/y=w760:dbl)
            n389 = Square Root(x=3.0) -> (sqrt(x)=w759:dbl)
            n390 = Divide(x=w760, y=w759) -> (x/y=w757:dbl)
            "Accuracy Reference Instrument (FS-2012)" <- w757
          }
          frame #4 {
            n391 = local read "Max Deviation"() -> (w767:dbl)
            n392 = Square Root(x=12.0) -> (sqrt(x)=w764:dbl)
            n393 = Divide(x=w767, y=w764) -> (x/y=w765:dbl)
            "Hysteresis Uncertainty" <- w765
          }
          frame #5 {
            n394 = local read "max value"() -> (w771:dbl)
            n395 = Square Root(x=3.0) -> (sqrt(x)=w770:dbl)
            n396 = Divide(x=w771, y=w770) -> (x/y=w768:dbl)
            "Uncertainty linearity error" <- w768
          }
          frame #6 {
            n397 = Build Array(w777, w776, w775, w773, w772) -> (w774:dbl[])
          }
          frame #7 {
            n398 = Square(x=w789) -> (x^2=w788:dbl[])
            n399 = Add Array Elements(numeric array=w788) -> (sum=w787:dbl)
            n400 = Square Root(x=w787) -> (sqrt(x)=w784:dbl)
            "Absolute Uncertainty" <- w784
            n401 = Divide(x=w784, y=10000.0) -> (x/y=w783:dbl)
            n402 = Multiply(x=w783, y=100.0) -> (x*y=w780:dbl)
            "Absolute Uncertainty in %FSO" <- w780
            n403 = Multiply(x=2.0, y=w780) -> (x*y=→"Expanded Uncertainty in %FSO":dbl)
            n404 = Multiply(x=2.0, y=w784) -> (x*y=→"Expanded Uncertainty":dbl)
          }
        }
      }
      frame "certificate" {
        n405 = stacked-sequence {
          seq-local: [w797 _ _ _ _ _ _ _ _] -> [_ _ _ _ w817 _ _ _ _]
          seq-local: [_ w802 _ _ _ _ _ _ _] -> [_ _ _ _ w822 _ _ _ _]
          seq-local: [_ _ w808 _ _ _ _ _ _] -> [_ _ _ _ w821 _ _ _ _]
          seq-local: [_ _ _ w812 _ _ _ _ _] -> [_ _ _ _ w820 _ _ _ _]
          seq-local: [_ _ _ _ w818 _ _ _ _] -> [_ _ _ _ _ _ _ _ w859]
          seq-local: [_ _ _ _ _ w823 _ _ _] -> [_ _ _ _ _ _ _ _ w860]
          seq-local: [_ _ _ _ _ _ w837 _ _] -> [_ _ _ _ _ _ _ _ w856]
          seq-local: [_ _ _ _ _ _ _ w846 _] -> [_ _ _ _ _ _ _ _ w852]
          frame #0 {
            n406 = local read "analog_salita_1"() -> (w793:dbl[][])
            n407 = local read "total_flow"() -> (w796:dbl[][])
            n408 = call "mead_and_deviation.vi"("insieme"=w796) -> ("Media"=w795:dbl[])  [unwired: 3 in, 1 out]
            n409 = call "mead_and_deviation.vi"("insieme"=w793) -> ("Media"=w794:dbl[])  [unwired: 3 in, 1 out]
            n410 = call "pbp_uncertainty.vi"("insieme"=w793) -> ("Incertezza"=w791:dbl[])  [unwired: 4 in]
            n411 = Multiply(x=w791, y=2.0) -> (x*y=w792:dbl[])
            n412 = Build Array(w795, w794, w792) -> (w797:dbl[][])
          }
          frame #1 {
            n413 = local read "analog_discesa_1"() -> (w798:dbl[][])
            n414 = call "pbp_uncertainty.vi"("insieme"=w798) -> ("Incertezza"=w799:dbl[])  [unwired: 4 in]
            n415 = call "mead_and_deviation.vi"("insieme"=w798) -> ("Media"=w803:dbl[])  [unwired: 3 in, 1 out]
            n416 = Multiply(x=w799, y=2.0) -> (x*y=w800:dbl[])
            n417 = Build Array(w803, w800) -> (w802:dbl[][])
          }
          frame #2 {
            n418 = local read "analog_salita_2"() -> (w804:dbl[][])
            n419 = call "pbp_uncertainty.vi"("insieme"=w804) -> ("Incertezza"=w806:dbl[])  [unwired: 4 in]
            n420 = call "mead_and_deviation.vi"("insieme"=w804) -> ("Media"=w809:dbl[])  [unwired: 3 in, 1 out]
            n421 = Multiply(x=w806, y=2.0) -> (x*y=w805:dbl[])
            n422 = Build Array(w809, w805) -> (w808:dbl[][])
          }
          frame #3 {
            n423 = local read "analog_discesa_2"() -> (w810:dbl[][])
            n424 = call "pbp_uncertainty.vi"("insieme"=w810) -> ("Incertezza"=w813:dbl[])  [unwired: 4 in]
            n425 = call "mead_and_deviation.vi"("insieme"=w810) -> ("Media"=w815:dbl[])  [unwired: 3 in, 1 out]
            n426 = Multiply(x=w813, y=2.0) -> (x*y=w811:dbl[])
            n427 = Build Array(w815, w811) -> (w812:dbl[][])
          }
          frame #4 {
            n428 = local read "Media"() -> (w816:dbl[])
            n429 = Build Array (concatenate)(w817, w822, w821, w820, w816) -> (w819:dbl[][])
            n430 = call "convert_table.vi"("Table Doubles"=w819) -> ("Table Strings"=w818:string[][])  [unwired: 10 in]
            "Table Strings" <- w818
          }
          frame #5 {
            n431 = local read "Arduino"() -> (w836:string)
            n432 = local read "DAQ"() -> (w835:string)
            n433 = local read "Air Pump"() -> (w834:string)
            n434 = local read "Description"() -> (w832:string)
            n435 = local read "Manufacturer"() -> (w824:string)
            n436 = local read "Series"() -> (w831:string)
            n437 = local read "Sensing Range"() -> (w830:string)
            n438 = local read "Operator"() -> (w829:string)
            n439 = local read "Temperature"() -> (w825:string)
            n440 = local read "Gas used"() -> (w828:string)
            n441 = local read "PSU A"() -> (w826:string)
            n442 = Bundle By Name(cluster=T14 {"Description"="", "Manufacturer"="", "Series"="", "Sensing Range"="", "Operator"="", "Temperature"="", "PSU A"="", "PSU B"="", "Gas used"="", "Air Pump"="", "DAQ"="", "Arduino"=""} ("Calibration Info"), "Arduino"=w836, "DAQ"=w835, "Air Pump"=w834, "Description"=w832, "Manufacturer"=w824, "Series"=w831, "Sensing Range"=w830, "Operator"=w829, "Temperature"=w825, "PSU A"=w826, "PSU B"="TTi QL355TP", "Gas used"=w828) -> (w823:T14)
          }
          frame #6 {
            n443 = local read "m avg"() -> (w845:dbl)
            n444 = local read "b avg"() -> (w842:dbl)
            n445 = Number To Fractional String(number=w845, precision (6)=i16 2) -> (F-format string=w839:string)  [unwired: 2 in]
            n446 = Number To Fractional String(number=w842, precision (6)=i16 1) -> (F-format string=w838:string)  [unwired: 2 in]
            n447 = Concatenate Strings("V = " ("string"), w839, "*F + " ("string"), w838) -> (w837:string)
          }
          frame #7 {
            n448 = local read "Absolute Uncertainty"() -> (w849:dbl)
            n449 = local read "Max Deviation"() -> (w851:dbl)
            n450 = local read "max value"() -> (w850:dbl)
            n451 = local read "Absolute Uncertainty in %FSO"() -> (w848:dbl)
            n452 = local read "Expanded Uncertainty in %FSO"() -> (w847:dbl)
            n453 = Build Array(w851, w850, w849, w848, w847) -> (w846:dbl[])
          }
          frame #8 {
            n454 = control-ref of="Calibration Curve"() -> (w857:refnum<vi>)
            n455 = local read "Base Programs Path"() -> (w858:path)
            n456 = control-ref of="Hysteresis Graph"() -> (w853:refnum<vi>)
            n457 = control-ref of="D 2"() -> (w854:refnum<vi>)
            n458 = control-ref of="A 2"() -> (w855:refnum<vi>)
            n459 = call "report.vi"("Calibration Info"=w860, "D"=w854, "A"=w855, "Absolute Uncertainties"=w852, "data"=w859, "H_a"=w853, "H_d"=w857, "Equation Asc."=w856, "path"=w858) -> ()  [unwired: 18 in, 1 out]
          }
        }
      }
      frame "simulate" {
        n460 = local read "Ring"() -> (w861:u16)
        n461 = stacked-sequence {
          seq-local: [w863 _ _ _ _ _ _] -> [_ _ _ w890 w895 w900 _]
          seq-local: [_ w872 _ _ _ _ _] -> [_ _ _ w889 w894 w899 _]
          seq-local: [_ _ w880 _ _ _ _] -> [_ _ _ w888 w893 w898 w902]
          tunnel: w861 -> [w862 w871 _ _ _ _ _]
          frame #0 {
            n462 = local read "Analog Salita"() -> (w864:dbl[][])
            n463 = case shown="1" w862 {
              tunnel: w864 -> [w867 w870]
              tunnel: [w865 w868] -> w863
              frame 1 {
                n464 = Array Subset(array=w867, length (row)=100 ("length")) -> (w865:dbl[][])  [unwired: 3 in]
              }
              frame 0, Default {
                n465 = Array Subset(array=w870, index (row)=100 ("length")) -> (w868:dbl[][])  [unwired: 3 in]
              }
            }
          }
          frame #1 {
            n466 = local read "Digital Salita"() -> (w873:dbl[][])
            n467 = case shown="1" w871 {
              tunnel: w873 -> [w876 w879]
              tunnel: [w874 w877] -> w872
              frame 1 {
                n468 = Array Subset(array=w876, length (row)=100 ("length")) -> (w874:dbl[][])  [unwired: 3 in]
              }
              frame 0, Default {
                n469 = Array Subset(array=w879, index (row)=100 ("length")) -> (w877:dbl[][])  [unwired: 3 in]
              }
            }
          }
          frame #2 {
            n470 = local read "index"() -> (w881:string)
            n471 = Decimal String To Number(string=w881) -> (number=w880:i32)  [unwired: 2 in, 1 out]
          }
          frame #3 {
            n472 = Index Array(array=w890, index (col)=w888) -> (element=w885:dbl[])  [unwired: 1 in]
            n473 = Index Array(array=w889, index (col)=w888) -> (element=w883:dbl[])  [unwired: 1 in]
            n474 = local write "Digital  Flow Sensor"(w883) -> ()
            n475 = local write "Analog  Flow Sensor"(w885) -> ()
            n476 = Index Array(array=w885, index=99) -> (element=w887:dbl)
            n477 = Index Array(array=w883, index=99) -> (element=w882:dbl)
            n478 = local write "volt"(w887) -> ()
            n479 = local write "flow"(w882) -> ()
          }
          frame #4 {
            n480 = Array Subset(array=w894, length (col)=w893) -> (w891:dbl[][])  [unwired: 3 in]
            n481 = Array Subset(array=w895, length (col)=w893) -> (w892:dbl[][])  [unwired: 3 in]
            n482 = local write "Analog Dataset"(w892) -> ()
            n483 = local write "Digital Dataset"(w891) -> ()
          }
          frame #5 {
            n484 = Index Array(array=w900, index (col)=w898) -> (element=w897:dbl[])  [unwired: 1 in]
            n485 = Index Array(array=w899, index (col)=w898) -> (element=w896:dbl[])  [unwired: 1 in]
            n486 = local write "Flow Rate (mL/min)"(w896) -> ()
            n487 = local write "Voltage (mV)"(w897) -> ()
          }
          frame #6 {
            n488 = local read "Input Sequence"() -> (w903:dbl[])
            n489 = Index Array(array=w903, index=w902) -> (element=w901:dbl)
            n490 = local write "output current"(w901) -> ()
          }
        }
      }
    }
  }
  n491 = while {
    tunnel: w10 -> [w921]
    tunnel: w11 -> [w918]
    shift-right: [w917] -> _
    shift-left: w14 -> [w916]
    tunnel: w2 -> [w913]
    stop <- w919 stop-if-true
    # "PRODUCER LOOP"
    n492 = event shown="[17] \"Ring\", \"index\", \"Histogram intervals\", \"Sensor & Phase\", \"Tab Control 5\": Value Change" {
      selector: _ -> [_ _ _ _ _ _ _ _ _ _ _ _ _ _ _ _ _ _ _ _ _ _ _ _]
      dyn-events: _ -> [_ _ _ _ _ _ _ _ _ _ _ _ _ _ _ _ _ _ _ _ _ _ _ _]
      timeout: _ -> [_ _ _ _ _ _ _ _ _ _ _ _ _ _ _ _ _ _ _ _ _ _ _ _]
      tunnel: w921 -> [w939 w970 w992 w994 w1009 _ w1052 _ _ _ _ _ _ w1104 _ _ _ _ w1156 _ _ w1181 _ _]
      tunnel: [w941 w967 w990 w993 w1008 w1043 w1050 _ w1076 _ w1091 _ _ w1103 _ w1121 _ w1125 w1155 w1158 w1178 w1186 _ w1188] -> w920
      tunnel: w918 -> [w938 w965 w987 w995 w1007 _ _ _ _ _ w1095 _ _ w1105 _ w1123 _ _ w1151 _ _ w1184 _ _]
      tunnel: w916 -> [w937 w968 w991 _ w1006 w1047 w1051 _ w1075 _ w1094 _ _ w1103 _ w1122 _ w1126 w1154 w1159 w1179 w1185 _ w1189]
      tunnel: [w933 w966 w988 _ w1005 _ _ _ _ _ _ _ _ w1104 _ _ _ _ w1152 _ _ w1181 _ _] -> w915
      tunnel: [w934 w964 w987 _ w1004 _ _ _ _ _ w1093 _ _ w1105 _ _ _ _ w1151 _ _ w1182 _ _] -> w914
      tunnel: w913 -> [_ _ _ _ _ w1048 _ _ w1078 _ _ _ _ _ _ _ _ w1127 _ w1160 w1180 _ _ w1191]
      event "POWER": Value Change {
        n493 = event-data() -> ()  [unwired: 1 in, 1 out]
        n494 = case shown="True" "POWER" {
          tunnel: [w944 w961] -> w940
          tunnel: w939 -> [w948 w963]
          tunnel: w938 -> [w945 _]
          tunnel: w937 -> [w947 w962]
          tunnel: [w946 _] -> w935
          tunnel: [w943 w959] -> w933
          tunnel: [w942 _] -> w934
          frame True {
            n495 = stacked-sequence {
              tunnel: w948 -> [w953 _]
              tunnel: w947 -> [w951 w958]
              tunnel: [_ w955] -> w946
              tunnel: w945 -> [_ w957]
              tunnel: [w950 _] -> w944
              tunnel: [w949 _] -> w943
              tunnel: [_ w954] -> w942
              frame #0 {
                # "initialize GPIB_USB"
                n496 = Enqueue Element(queue=w953, element=gpibusb."INIT", error in (no error)=w951) -> (queue out=w949:refnum<queue>, error out=w950:errorcluster)  [unwired: 1 in, 1 out]
              }
              frame #1 {
                # "initialize DAQ"
                n497 = Enqueue Element(queue=w957, element=daq."INIT", error in (no error)=w958) -> (queue out=w954:refnum<queue>, error out=w955:errorcluster)  [unwired: 1 in, 1 out]
              }
            }
          }
          frame False {
            # "initialize GPIB_USB"
            n498 = Enqueue Element(queue=w963, element=gpibusb."SHUTDOWN", error in (no error)=w962) -> (queue out=w959:refnum<queue>, error out=w961:errorcluster)  [unwired: 1 in, 1 out]
          }
        }
        n499 = Merge Errors(w940, w935) -> (w941:errorcluster)
      }
      event "Control Panel.Enable": Value Change {
        n500 = event-data() -> ("NewVal"=w969:bool)  [unwired: 1 in]
        n501 = case shown="True" w969 {
          tunnel: w970 -> [w978 w986]
          tunnel: w968 -> [w977 w985]
          tunnel: [w973 w984] -> w967
          tunnel: [w974 w982] -> w966
          tunnel: w965 -> [w975 w981]
          tunnel: [w975 w981] -> w964
          frame True {
            # "ENABLE current ramp procedure and\n ENABLE power supply output"
            n502 = local read "Control Panel"() -> (w972:T3)
            n503 = Unbundle By Name(w972) -> ("Start [mA]"=w971:i32)
            n504 = Enqueue Element(queue=w978, element=gpibusb."START", error in (no error)=w977) -> (queue out=w974:refnum<queue>, error out=w973:errorcluster)  [unwired: 1 in, 1 out]
            n505 = local write "output current"(w971) -> ()
          }
          frame False {
            # "DISABLE current ramp procedure and\n DISABLE power suplly's output"
            n506 = local read "Control Panel"() -> (w980:T3)
            n507 = Unbundle By Name(w980) -> ("Start [mA]"=w979:i32)
            n508 = Enqueue Element(queue=w986, element=gpibusb."STOP", error in (no error)=w985) -> (queue out=w982:refnum<queue>, error out=w984:errorcluster)  [unwired: 1 in, 1 out]
            n509 = local write "output current"(w979) -> ()
          }
        }
      }
      event "Control Panel.Step [mA]": Value Change {
        n510 = event-data() -> ()  [unwired: 1 in, 1 out]
        n511 = Enqueue Element(queue=w992, element=gpibusb."STEP", error in (no error)=w991) -> (queue out=w988:refnum<queue>, error out=w990:errorcluster)  [unwired: 1 in, 1 out]
      }
      event "Control Panel.Next": Value Change {
        n512 = event-data() -> ()  [unwired: 1 in, 1 out]
        n513 = stacked-sequence {
          tunnel: w995 -> [w997 _ _]
          tunnel: w994 -> [_ w999 w1002]
          tunnel: [_ _ w1000] -> w993
          frame #0 {
            n514 = Enqueue Element(queue=w997, element=daq."FLUSH") -> ()  [unwired: 2 in, 3 out]
          }
          frame #1 {
            n515 = Enqueue Element(queue=w999, element=gpibusb."NEXT") -> ()  [unwired: 2 in, 3 out]
          }
          frame #2 {
            n516 = Enqueue Element(queue=w1002, element=gpibusb."CURR?") -> (error out=w1000:errorcluster)  [unwired: 2 in, 2 out]
          }
        }
      }
      event "Read": Value Change {
        n517 = event-data() -> ()  [unwired: 1 in, 1 out]
        n518 = case shown="True" "Read" {
          tunnel: w1009 -> [w1014 w1030]
          tunnel: [w1010 w1026] -> w1008
          tunnel: w1007 -> [w1015 w1031]
          tunnel: w1006 -> [w1013 w1029]
          tunnel: [w1012 w1028] -> w1005
          tunnel: [w1011 w1027] -> w1004
          frame True {
            # "Start Acquisition Samples (Both Flow Sensors)"
            n519 = stacked-sequence {
              tunnel: w1015 -> [_ w1024 _]
              tunnel: w1014 -> [w1020 _ _]
              tunnel: w1013 -> [w1019 w1022 _]
              tunnel: [w1018 _ _] -> w1012
              tunnel: [_ w1023 _] -> w1011
              tunnel: [w1016 _ _] -> w1010
              frame #0 {
                n520 = Enqueue Element(queue=w1020, element=gpibusb."READ_DIGITAL", error in (no error)=w1019) -> (queue out=w1018:refnum<queue>, error out=w1016:errorcluster)  [unwired: 1 in, 1 out]
              }
              frame #1 {
                n521 = Enqueue Element(queue=w1024, element=daq."READ_VOLTAGE", error in (no error)=w1022) -> (queue out=w1023:refnum<queue>)  [unwired: 1 in, 2 out]
              }
              frame #2 {
                n522 = property on="Samples" class="DigNum (strict)"("DisabledEnum"=T13."Disabled and Grayed Out" ("Disabled")) -> ()  [unwired: 2 in, 2 out]
              }
            }
          }
          frame False {
            # "Stop Acquisition Samples"
            n523 = stacked-sequence {
              tunnel: w1031 -> [_ w1040 _]
              tunnel: w1030 -> [w1036 _ _]
              tunnel: w1029 -> [w1035 w1038 _]
              tunnel: [w1034 _ _] -> w1028
              tunnel: [_ w1039 _] -> w1027
              tunnel: [w1032 _ _] -> w1026
              frame #0 {
                # "(idle)"
                n524 = Enqueue Element(queue=w1036, element=gpibusb."READ_DIGITAL", error in (no error)=w1035) -> (queue out=w1034:refnum<queue>, error out=w1032:errorcluster)  [unwired: 1 in, 1 out]
              }
              frame #1 {
                n525 = Enqueue Element(queue=w1040, element=daq."CLEAR", error in (no error)=w1038) -> (queue out=w1039:refnum<queue>)  [unwired: 1 in, 2 out]
              }
              frame #2 {
                n526 = property on="Samples" class="DigNum (strict)"("DisabledEnum"=T13."Enabled" ("Disabled")) -> ()  [unwired: 2 in, 2 out]
              }
            }
          }
        }
      }
      event "calibrate!": Value Change {
        n527 = event-data() -> ()  [unwired: 1 in, 1 out]
        n528 = Enqueue Element(queue=w1048, element=calib."combined uncertainty", error in (no error)=w1047) -> (queue out=w1046:refnum<queue>, error out=w1045:errorcluster)  [unwired: 1 in, 1 out]
        n529 = Enqueue Element(queue=w1046, element=calib."certificate", error in (no error)=w1045) -> (error out=w1043:errorcluster)  [unwired: 1 in, 2 out]
      }
      event "Sampling Frequency (Hz)": Value Change {
        n530 = event-data() -> ()  [unwired: 1 in, 1 out]
        n531 = Enqueue Element(queue=w1052, element=gpibusb."FREQ", error in (no error)=w1051) -> (error out=w1050:errorcluster)  [unwired: 1 in, 2 out]
      }
      event "DATASET_STORE": Value Change {
        n532 = event-data() -> ()  [unwired: 1 in, 1 out]
        n533 = stacked-sequence {
          tunnel: "Phase" -> [w1063 w1069]
          tunnel: "Ring 2" -> [w1062 w1066]
          tunnel: [_ w1068] -> w1055
          tunnel: [w1061 _] -> _
          tunnel: [w1060 _] -> w1053
          tunnel: [_ w1067] -> w1054
          frame #0 {
            n534 = local read "Digital Dataset"() -> (w1058:dbl[][])
            n535 = call "append to file.vi"("Analog Dataset"=w1058, "Ring 2"=w1062, "Phase"=w1063, "file path (use dialog)"="Dataset D Digital") -> ("error out"=w1061:errorcluster, "output string"=w1060:string)
          }
          frame #1 {
            n536 = local read "Analog Dataset"() -> (w1065:dbl[][])
            n537 = call "append to file.vi"("Analog Dataset"=w1065, "Ring 2"=w1066, "Phase"=w1069, "file path (use dialog)"="Dataset A Path") -> ("error out"=w1068:errorcluster, "output string"=w1067:string)
          }
        }
        n538 = case shown="No Error" w1055 {
          tunnel: w1054 -> [w1072 _]
          tunnel: w1053 -> [w1070 _]
          frame No Error {
            n539 = Concatenate Strings(w1072, "\n" ("string"), w1070) -> (w1073:string)
            n540 = One Button Dialog(message=w1073) -> ()  [unwired: 1 in, 1 out]
          }
          frame Error {
            n541 = One Button Dialog(message="Oops!") -> ()  [unwired: 1 in, 1 out]
          }
        }
      }
      event "Load Files": Value Change {
        n542 = event-data() -> ()  [unwired: 1 in, 1 out]
        n543 = Enqueue Element(queue=w1078, element=calib."load_measures", error in (no error)=w1075) -> (error out=w1076:errorcluster)  [unwired: 1 in, 2 out]
      }
      event "Save": Value Change {
        n544 = event-data() -> ()  [unwired: 1 in, 1 out]
        n545 = local read "Voltage (mV)"() -> (w1079:dbl[])
        n546 = Array Size(array=w1079) -> (size(s)=w1080:i32)
        n547 = stacked-sequence {
          tunnel: w1080 -> [_ w1085]
          tunnel: w1079 -> [w1081 _]
          frame #0 {
            n548 = local read "Analog Dataset"() -> (w1082:dbl[][])
            n549 = Matrix Size(0:w1082) -> (2:w1083:i32)  [unwired: 1 out]
            n550 = Insert Into Array(array=w1082, index (col)=w1083, new element=w1081) -> (w1084:dbl[][])  [unwired: 1 in]
            n551 = local write "Analog Dataset"(w1084) -> ()
          }
          frame #1 {
            n552 = local read "Flow Rate (mL/min)"() -> (w1087:dbl[])
            n553 = local read "Digital Dataset"() -> (w1088:dbl[][])
            n554 = Matrix Size(0:w1088) -> (2:w1089:i32)  [unwired: 1 out]
            n555 = Array Subset(array=w1087, length=w1085) -> (w1086:dbl[])  [unwired: 1 in]
            n556 = Insert Into Array(array=w1088, index (col)=w1089, new element=w1086) -> (w1090:dbl[][])  [unwired: 1 in]
            n557 = local write "Digital Dataset"(w1090) -> ()
          }
        }
      }
      event "POWER 2": Value Change {
        n558 = event-data() -> ()  [unwired: 1 in, 1 out]
        n559 = Enqueue Element(queue=w1095, element=daq."SHUTDOWN", error in (no error)=w1094) -> (queue out=w1093:refnum<queue>, error out=w1091:errorcluster)  [unwired: 1 in, 1 out]
      }
      event "POWER 3": Value Change {
        n560 = event-data() -> ()  [unwired: 1 in, 4 out]
        n561 = local read "POWER 3"() -> (w1096:bool)
        n562 = case shown="False" w1096 {
          frame False {
            n563 = Stop(stop? (T)=TRUE) -> ()
          }
          frame True {
            n564 = Stop(stop? (T)=FALSE) -> ()
          }
        }
      }
      event "Features": Value Change {
        # "update histogram interval values"
        n565 = event-data() -> ()  [unwired: 1 in, 4 out]
        n566 = local read "Features"() -> (w1102:i32)
        n567 = local read "Control Panel"() -> (w1101:T3)
        n568 = Unbundle By Name(w1101) -> ("Start [mA]"=w1100:i32, "Step [mA]"=w1099:i32)
        n569 = call "inout.vi"("Step [mA]"=w1099, "Initial Value [mA]"=w1100, "# Steps"=w1102) -> ()  [unwired: 8 in, 1 out]
      }
      event "CLEAR BUTTON": Value Change {
        n570 = event-data() -> ()  [unwired: 1 in, 1 out]
        n571 = stacked-sequence {
          frame #0 {
            n572 = local write "Digital Discesa"(dbl[][] []) -> ()
            n573 = local write "Digital Salita"(dbl[][] []) -> ()
          }
          frame #1 {
            n574 = local write "Analog Discesa"(dbl[][] []) -> ()
            n575 = local write "Analog Salita"(dbl[][] []) -> ()
          }
        }
      }
      event "Scale Voltage", "Scale Flow": Value Change {
        n576 = event-data() -> ()  [unwired: 1 in, 1 out]
        n577 = stacked-sequence {
          frame #0 {
            n578 = case shown="\"(mV)\"" "Scale Voltage" {
              frame "(mV)" {
                n579 = local write "scale_analog"(1000.0 ("scale_digital")) -> ()
              }
              frame "(V)", Default {
                n580 = local write "scale_analog"(1.0) -> ()
              }
            }
            n581 = Concatenate Strings("Voltage " ("string"), "Scale Voltage") -> (w1110:string)
            n582 = property on="Analog  Flow Sensor" class="WFGraph (strict)"("YScale.NameLbl.Text"=w1110) -> ()  [unwired: 2 in, 2 out]
          }
          frame #1 {
            n583 = case shown="\"(mL/min)\"" "Scale Flow" {
              frame "(mL/min)" {
                n584 = local write "scale_digital"(1000.0 ("scale_digital")) -> ()
              }
              frame "(L/min)", Default {
                n585 = local write "scale_digital"(1.0) -> ()
              }
            }
            n586 = Concatenate Strings("Flow Rate " ("string"), "Scale Flow") -> (w1117:string)
            n587 = property on="Digital  Flow Sensor" class="WFGraph (strict)"("YScale.NameLbl.Text"=w1117) -> ()  [unwired: 2 in, 2 out]
          }
        }
      }
      event "Sampling Rate (Sa/s)", "Buffer Size (Sa)": Value Change {
        n588 = event-data() -> ()  [unwired: 1 in, 1 out]
        n589 = Enqueue Element(queue=w1123, element=daq."PARAMETERS", error in (no error)=w1122) -> (error out=w1121:errorcluster)  [unwired: 1 in, 2 out]
      }
      event "Base Programs Path": Value Change {
        # "to be implemented."
        n590 = event-data() -> ()  [unwired: 1 in, 1 out]
      }
      event "Ring", "index", "Histogram intervals", "Sensor & Phase", "Tab Control 5": Value Change {
        n591 = event-data() -> ()  [unwired: 1 in, 1 out]
        n592 = stacked-sequence {
          tunnel: w1127 -> [_ _ w1139 w1142 w1146 w1149]
          tunnel: w1126 -> [_ _ w1138 w1141 w1145 w1148]
          tunnel: [_ _ _ _ _ w1147] -> w1125
          tunnel: [w1128 _ _ _ _ _] -> w1124
          tunnel: [_ w1134 _ _ _ _] -> _
          frame #0 {
            n593 = local read "Sensor & Phase"() -> (w1129:T4)
            n594 = case shown="\"Analog (Increasing Values)\"" w1129 {
              tunnel: ["Voltage (mV)" ("Y Scale.Name Label.Text") "Voltage (mV)" ("Y Scale.Name Label.Text") "Flow (mL/min)" ("Y Scale.Name Label.Text") "Flow (mL/min)" ("Y Scale.Name Label.Text")] -> w1128
              frame "Analog (Increasing Values)" {
              }
              frame "Analog (Decreasing Values)" {
              }
              frame "Digital (Decreasing Values)" {
              }
              frame "Digital (Increasing Values)" {
              }
            }
          }
          frame #1 {
            n595 = local read "Tab Control 5"() -> (w1135:T6)
            n596 = case shown="\" Descending\"" w1135 {
              tunnel: ["Voltage (mV)" ("Y Scale.Name Label.Text") "Flow (mL/min)" ("Y Scale.Name Label.Text")] -> w1134
              frame " Ascending", Default {
              }
              frame " Descending" {
              }
            }
          }
          frame #2 {
            n597 = Enqueue Element(queue=w1139, element=calib."boxplot", error in (no error)=w1138) -> ()  [unwired: 1 in, 3 out]
          }
          frame #3 {
            n598 = Enqueue Element(queue=w1142, element=calib."histogram", error in (no error)=w1141) -> ()  [unwired: 1 in, 3 out]
          }
          frame #4 {
            n599 = Enqueue Element(queue=w1146, element=calib."combined uncertainty", error in (no error)=w1145) -> ()  [unwired: 1 in, 3 out]
          }
          frame #5 {
            n600 = Enqueue Element(queue=w1149, element=calib."results", error in (no error)=w1148) -> (error out=w1147:errorcluster)  [unwired: 1 in, 2 out]
          }
        }
        n601 = property on="Box Plot" class="XYGraph (strict)"("YScale.NameLbl.Text"=w1124) -> ()  [unwired: 2 in, 2 out]
        n602 = property on="Histogram" class="XYGraph (strict)"("XScale.NameLbl.Text"=w1124) -> ()  [unwired: 2 in, 2 out]
      }
      event "serial port": Value Change {
        n603 = event-data() -> ()  [unwired: 1 in, 1 out]
        n604 = Enqueue Element(queue=w1156, element=gpibusb."ARDUINO_SETTINGS", error in (no error)=w1154) -> (queue out=w1152:refnum<queue>, error out=w1155:errorcluster)  [unwired: 1 in, 1 out]
      }
      event "Tab Control 9": Value Change {
        n605 = event-data() -> ()  [unwired: 1 in, 1 out]
        n606 = local read "Tab Control 9"() -> (w1157:T9)
        n607 = case shown="\"Ascending (Flow in vs. Flow Out)\"" w1157 {
          tunnel: w1160 -> [w1164 w1168 w1172 w1176]
          tunnel: w1159 -> [w1162 w1166 w1171 w1175]
          tunnel: [w1161 w1165 w1170 w1174] -> w1158
          frame "Ascending (Voltage vs. Flow)", Default {
            n608 = Enqueue Element(queue=w1164, element=calib."linear regression", error in (no error)=w1162) -> (error out=w1161:errorcluster)  [unwired: 1 in, 2 out]
          }
          frame "Descending (Voltage vs. Flow)" {
            n609 = Enqueue Element(queue=w1168, element=calib."linear regression", error in (no error)=w1166) -> (error out=w1165:errorcluster)  [unwired: 1 in, 2 out]
          }
          frame "Descending (Flow in vs. Flow out)" {
            n610 = Enqueue Element(queue=w1172, element=calib."linearization", error in (no error)=w1171) -> (error out=w1170:errorcluster)  [unwired: 1 in, 2 out]
          }
          frame "Ascending (Flow in vs. Flow Out)" {
            n611 = Enqueue Element(queue=w1176, element=calib."linearization", error in (no error)=w1175) -> (error out=w1174:errorcluster)  [unwired: 1 in, 2 out]
          }
        }
      }
      event "Plot": Value Change {
        n612 = event-data() -> ()  [unwired: 1 in, 6 out]
        n613 = Enqueue Element(queue=w1180, element=calib."calibration curve", error in (no error)=w1179) -> (error out=w1178:errorcluster)  [unwired: 1 in, 2 out]
      }
      event "Channel": Value Change {
        n614 = event-data() -> ()  [unwired: 1 in, 1 out]
        n615 = Enqueue Element(queue=w1184, element=daq."DAQ_SETTINGS", error in (no error)=w1185) -> (queue out=w1182:refnum<queue>, error out=w1186:errorcluster)  [unwired: 1 in, 1 out]
      }
      event "DATASET_CLEAR": Value Change {
        w1187 = dbl[][] []
        n616 = event-data() -> ()  [unwired: 1 in, 1 out]
        n617 = local write "Digital Dataset"(w1187) -> ()
        n618 = local write "Analog Dataset"(w1187) -> ()
      }
      event "Plot Signals": Value Change {
        n619 = event-data() -> ()  [unwired: 1 in, 1 out]
        n620 = Enqueue Element(queue=w1191, element=calib."simulate", error in (no error)=w1189) -> (error out=w1188:errorcluster)  [unwired: 1 in, 2 out]
      }
    }
    n621 = case shown="No Error" w920 {
      selector: w920 -> [w922 w927]
      tunnel: [FALSE FALSE] -> w919
      tunnel: [w922 w926] -> w917
      tunnel: w915 -> [_ w931]
      tunnel: w914 -> [_ w930]
      frame No Error {
      }
      frame Error {
        n622 = Enqueue Element(queue=w931, element=gpibusb."ERROR", error in (no error)=w927) -> (error out=w925:errorcluster)  [unwired: 1 in, 2 out]
        n623 = Enqueue Element(queue=w930, element=daq."ERROR", error in (no error)=w927) -> (error out=w924:errorcluster)  [unwired: 1 in, 2 out]
        n624 = Merge Errors(w925, w924) -> (w926:errorcluster)
      }
    }
    n625 = Wait Until Next ms Multiple(millisecond multiple=u32 10) -> ()  [unwired: 1 out]
  }
  n626 = while {
    tunnel: w10 -> [w1210]
    shift-right: [w1204] -> _
    shift-left: w9 -> [w1209]
    shift-right: [w1202] -> _
    shift-left: dbl[] [] -> [w1203]
    shift-right: [w1200] -> _
    shift-left: _ -> [w1195]
    shift-right: [w1201] -> _
    shift-left: _ -> [w1194]
    shift-right: [w1198] -> _
    shift-left: _ -> [w1197]
    stop <- w1207 stop-if-true
    # "ARDUINO & POWER SUPPLY CONTROLS CONSUMER LOOP"
    n627 = case shown="No Error" w1209 {
      selector: w1209 -> [w1217 w1223]
      tunnel: w1210 -> [w1218 w1224]
      tunnel: [w1216 w1224] -> w1206
      tunnel: [w1215 w1223] -> w1205
      tunnel: [w1212 w1222] -> w1192
      tunnel: w1194 -> [w1212 w1222]
      tunnel: [w1213 w1221] -> w1193
      tunnel: w1195 -> [w1213 w1221]
      tunnel: [w1214 gpibusb."ERROR" ("element")] -> w1199
      tunnel: [w1211 w1219] -> w1196
      tunnel: w1197 -> [w1211 w1219]
      frame No Error {
        # "Guard Clause"
        n628 = Dequeue Element(queue=w1218, error in (no error)=w1217) -> (queue out=w1216:refnum<queue>, element=w1214:T11, error out=w1215:errorcluster)  [unwired: 1 in, 1 out]
      }
      frame Error {
        # "Guard Clause"
      }
    }
    n629 = case shown="\"READ_DIGITAL\"" w1199 {
      tunnel: [FALSE _ _ _ _ _ _ _ _ _ FALSE _] -> w1207
      tunnel: w1206 -> [_ _ w1291 w1314 _ _ _ _ _ _ _ _]
      tunnel: w1205 -> [w1225 w1263 w1289 w1316 w1345 w1356 w1365 w1372 w1388 w1394 w1410 w1418]
      tunnel: [w1226 w1265 w1288 w1317 w1346 w1355 w1364 w1368 w1389 w1393 w1414 w1422] -> w1204
      tunnel: w1203 -> [_ _ _ w1313 _ _ _ _ _ _ _ _]
      tunnel: [_ _ _ w1312 _ _ _ _ _ _ _ _] -> w1202
      tunnel: [w1228 w1267 w1286 w1309 w1347 w1350 w1358 w1367 w1386 w1397 w1412 w1420] -> w1201
      tunnel: [w1229 w1262 w1284 w1310 w1343 w1351 w1360 w1369 w1385 w1392 w1411 w1421] -> w1200
      tunnel: w1193 -> [_ w1264 w1290 w1310 w1348 w1357 w1366 w1371 w1385 w1395 w1411 w1419]
      tunnel: w1192 -> [_ w1267 w1286 w1315 w1347 w1350 w1358 w1367 w1386 w1397 w1412 w1420]
      tunnel: [w1227 w1266 w1285 w1311 w1342 w1349 w1359 w1370 w1387 w1396 w1413 w1417] -> w1198
      tunnel: w1196 -> [_ w1266 w1285 w1311 w1342 w1349 w1359 w1370 w1391 w1396 w1413 w1417]
      frame "INIT", Default {
        n630 = local read "Base Programs Path"() -> (w1230:path)
        n631 = stacked-sequence {
          seq-local: [w1234 _ _ _ _ _ _ _ _] -> [_ _ _ _ _ w1247 _ _ _]
          seq-local: [_ w1238 _ _ _ _ _ _ _] -> [_ _ _ _ _ _ w1254 _ w1261]
          seq-local: [_ _ w1240 _ _ _ _ _ _] -> [_ _ _ _ _ _ w1251 _ w1260]
          seq-local: [_ _ _ w1242 _ _ _ _ _] -> [_ _ _ _ _ _ w1252 _ w1259]
          seq-local: [_ _ _ _ _ w1246 _ _ _] -> [_ _ _ _ _ _ w1255 w1256 _]
          tunnel: w1230 -> [w1235 _ _ _ _ _ w1250 _ _]
          tunnel: "gpib address" -> [_ _ _ _ _ _ w1253 _ _]
          tunnel: [_ _ _ _ _ _ _ w1258 _] -> w1226
          tunnel: [_ _ _ _ _ _ _ _ w1261] -> w1229
          tunnel: [_ _ _ _ _ _ _ _ w1260] -> w1228
          tunnel: [_ _ _ _ _ _ _ _ w1259] -> w1227
          tunnel: w1225 -> [_ _ _ _ _ w1245 _ w1257 _]
          frame #0 {
            # "compose program path"
            n632 = Path To String(path=w1235) -> (string=w1237:string)
            n633 = Concatenate Strings(w1237, "\\labview\\Arduino_FlowPump_Controller.vi" ("string")) -> (w1236:string)
            n634 = String To Path(string=w1236) -> (path=w1234:path)
          }
          frame #1 {
            n635 = Obtain Queue(element data type="") -> (queue out=w1238:refnum<queue>)  [unwired: 4 in, 2 out]
          }
          frame #2 {
            n636 = Obtain Queue(element data type="") -> (queue out=w1240:refnum<queue>)  [unwired: 4 in, 2 out]
          }
          frame #3 {
            n637 = Obtain Queue(element data type="") -> (queue out=w1242:refnum<queue>)  [unwired: 4 in, 2 out]
          }
          frame #4 {
            w1244 = TRUE ("Boolean 5")
            "ARDUINO ON|OFF 2" <- w1244
            "POWER_SUPPLY ON|OFF 2" <- w1244
            "FS-2012 ON|OFF 2" <- w1244
          }
          frame #5 {
            n638 = vi-ref "GPIB_UART.lvlib:Arduino_FlowPump_Controller.vi"() -> (w1249:refnum<vi>)
            n639 = Open VI Reference(type specifier VI Refnum (for type only)=w1249, vi path=w1247, options=128, error in (no error)=w1245) -> (vi reference=w1246:refnum<vi>)  [unwired: 2 in, 1 out]
          }
          frame #6 {
            n640 = call-by-ref "Start Asynchronous Call"(reference=w1255, "commands"=w1254, "GPIB ADDRESS"=w1253, "DECODER_DATA"=w1252, "measurements"=w1251, "Base Path"=w1250) -> ()  [unwired: 7 in, 2 out]
          }
          frame #7 {
            n641 = invoke on="DIGITAL SENSOR  & POWER SUPPLY" class="SubPnl" method="Insert VI"(error in=w1257, "VI Ref"=w1256) -> (error out=w1258:errorcluster)  [unwired: 2 in, 3 out]
          }
          frame #8 {
          }
        }
      }
      frame "START" {
        n642 = stacked-sequence {
          seq-local: [_ w1271 _] -> [_ _ w1279]
          seq-local: [_ w1272 _] -> [_ _ w1278]
          tunnel: [_ _ w1280] -> w1265
          tunnel: w1264 -> [_ _ w1275]
          tunnel: w1263 -> [_ _ w1277]
          tunnel: [_ _ w1276] -> w1262
          frame #0 {
            n643 = local read "Control Panel"() -> (w1270:T3)
            n644 = Unbundle By Name(w1270) -> ("Start [mA]"=→"start_":i32, "Step [mA]"=→"step_":i32)
          }
          frame #1 {
            n645 = local read "start_"() -> (w1274:i32)
            n646 = local read "step_"() -> (w1273:i32)
            n647 = Number To Decimal String(number=w1274) -> (decimal integer string=w1271:string)  [unwired: 1 in]
            n648 = Number To Decimal String(number=w1273) -> (decimal integer string=w1272:string)  [unwired: 1 in]
          }
          frame #2 {
            # "WRITES COMMAND\nE.G., START:250:25"
            n649 = Concatenate Strings("START:" ("element"), w1279, ":" ("string"), w1278) -> (w1283:string)
            n650 = Enqueue Element(queue=w1275, element=w1283, error in (no error)=w1277) -> (queue out=w1276:refnum<queue>, error out=w1280:errorcluster)  [unwired: 1 in, 1 out]
          }
        }
      }
      frame "READ_DIGITAL" {
        n651 = local read "Read"() -> (w1287:bool)
        n652 = case shown="True" w1287 {
          tunnel: w1291 -> [w1296 _]
          tunnel: w1290 -> [w1295 w1308]
          tunnel: [w1292 w1306] -> w1284
          tunnel: w1289 -> [w1293 w1305]
          tunnel: [w1294 w1304] -> w1288
          frame True {
            n653 = stacked-sequence {
              tunnel: w1296 -> [_ w1302]
              tunnel: w1295 -> [w1301 _]
              tunnel: [w1299 _] -> w1294
              tunnel: w1293 -> [w1298 _]
              tunnel: [w1297 _] -> w1292
              frame #0 {
                n654 = Enqueue Element(queue=w1301, element="READ_ARDUINO", error in (no error)=w1298) -> (queue out=w1297:refnum<queue>, error out=w1299:errorcluster)  [unwired: 1 in, 1 out]
              }
              frame #1 {
                n655 = Enqueue Element(queue=w1302, element=gpibusb."ACQUIRE") -> ()  [unwired: 2 in, 3 out]
              }
            }
          }
          frame False {
            n656 = Enqueue Element(queue=w1308, element="READ_ALL:0", error in (no error)=w1305) -> (queue out=w1306:refnum<queue>, error out=w1304:errorcluster)  [unwired: 1 in, 1 out]
          }
        }
      }
      frame "ACQUIRE" {
        n657 = stacked-sequence {
          seq-local: [w1323 _ _] -> [_ _ w1332]
          seq-local: [w1321 _ _] -> [_ w1329 _]
          tunnel: w1313 -> [w1326 _ _]
          tunnel: w1315 -> [w1325 _ _]
          tunnel: w1316 -> [w1324 _ _]
          tunnel: w1314 -> [_ _ w1330]
          tunnel: [w1322 _ _] -> w1309
          tunnel: [_ _ w1331] -> w1317
          tunnel: [_ w1329 _] -> w1312
          frame #0 {
            # "FETCH"
            n658 = Dequeue Element(queue=w1325, error in (no error)=w1324) -> (queue out=w1322:refnum<queue>, element=w1327:string, error out=w1323:errorcluster)  [unwired: 1 in, 1 out]
            n659 = Fract/Exp String To Number(use system decimal point (T)=FALSE, string=w1327) -> (number=w1319:dbl)  [unwired: 2 in, 1 out]
            n660 = Multiply(x="scale_digital", y=w1319) -> (x*y=w1318:dbl)
            n661 = Build Array (concatenate)(w1326, w1318) -> (w1321:dbl[])
            n662 = local write "flow"(w1318) -> ()
          }
          frame #1 {
            # "update indicators"
            "Flow Rate (mL/min)" <- w1329
            "Digital  Flow Sensor" <- w1329
          }
          frame #2 {
            n663 = local read "Read"() -> (w1333:bool)
            n664 = case shown="True" w1333 {
              tunnel: [w1337 w1339] -> w1331
              tunnel: w1330 -> [w1336 w1341]
              tunnel: w1332 -> [w1335 w1340]
              frame True {
                # "NEXT STATE\nTRANSITION"
                n665 = Enqueue Element(queue=w1336, element=gpibusb."ACQUIRE", error in (no error)=w1335) -> (error out=w1337:errorcluster)  [unwired: 1 in, 2 out]
              }
              frame False {
                # "(idle)"
                n666 = Enqueue Element(queue=w1341, element=gpibusb."READ_DIGITAL", error in (no error)=w1340) -> (error out=w1339:errorcluster)  [unwired: 1 in, 2 out]
              }
            }
          }
        }
      }
      frame "STOP" {
        # "STOP CALIBRATION PROCEDURE.\nDISABLE CURRENT RAMP\nDISABLE POWER SUPPLY OUTPUT"
        n667 = Enqueue Element(queue=w1348, element="STOP", error in (no error)=w1345) -> (queue out=w1343:refnum<queue>, error out=w1346:errorcluster)  [unwired: 1 in, 1 out]
      }
      frame "ARDUINO_SETTINGS" {
        n668 = Concatenate Strings("SET_PORT:" ("State"), "serial port") -> (w1352:string)
        n669 = Enqueue Element(queue=w1357, element=w1352, error in (no error)=w1356) -> (queue out=w1351:refnum<queue>, error out=w1355:errorcluster)  [unwired: 1 in, 1 out]
      }
      frame "FREQ" {
        n670 = Concatenate Strings("SF:" ("State"), "Sampling Frequency (Hz)") -> (w1361:string)
        n671 = Enqueue Element(queue=w1366, element=w1361, error in (no error)=w1365) -> (queue out=w1360:refnum<queue>, error out=w1364:errorcluster)  [unwired: 1 in, 1 out]
      }
      frame "NEXT" {
        n672 = stacked-sequence {
          seq-local: [w1375 _] -> [_ w1383]
          seq-local: [w1374 _] -> [_ w1381]
          tunnel: w1372 -> [w1377 _]
          tunnel: w1371 -> [w1376 _]
          tunnel: [_ w1380] -> w1369
          tunnel: [_ w1379] -> w1368
          frame #0 {
            n673 = Enqueue Element(queue=w1376, element="RAMP_NEXT", error in (no error)=w1377) -> (queue out=w1375:refnum<queue>, error out=w1374:errorcluster)  [unwired: 1 in, 1 out]
            n674 = Wait Until Next ms Multiple(millisecond multiple=u32 10) -> ()  [unwired: 1 out]
          }
          frame #1 {
            n675 = Enqueue Element(queue=w1383, element="CURR?", error in (no error)=w1381) -> (queue out=w1380:refnum<queue>, error out=w1379:errorcluster)  [unwired: 1 in, 1 out]
          }
        }
      }
      frame "CURR?" {
        n676 = Dequeue Element(queue=w1391, error in (no error)=w1388) -> (queue out=w1387:refnum<queue>, element=w1390:string, error out=w1389:errorcluster)  [unwired: 1 in, 1 out]
        n677 = Fract/Exp String To Number(string=w1390) -> (number=w1384:dbl)  [unwired: 3 in, 1 out]
        n678 = local write "output current"(w1384) -> ()
      }
      frame "STEP" {
        n679 = stacked-sequence {
          seq-local: [w1398 _ _ _] -> [_ w1401 _ _]
          seq-local: [_ w1400 _ _] -> [_ _ w1403 _]
          seq-local: [_ _ w1402 _] -> [_ _ _ w1407]
          tunnel: w1395 -> [_ _ _ w1409]
          tunnel: w1394 -> [_ _ _ w1408]
          tunnel: [_ _ _ w1406] -> w1393
          tunnel: [_ _ _ w1405] -> w1392
          frame #0 {
            n680 = local read "Control Panel"() -> (w1399:T3)
            n681 = Unbundle By Name(w1399) -> ("Step [mA]"=w1398:i32)
          }
          frame #1 {
            n682 = Number To Decimal String(number=w1401) -> (decimal integer string=w1400:string)  [unwired: 1 in]
          }
          frame #2 {
            n683 = call "conc_state_args.vi"("State"="RAMP_STEP", "Args"=w1403) -> ("state_and_args"=w1402:string)  [unwired: 13 in]
          }
          frame #3 {
            n684 = Enqueue Element(queue=w1409, element=w1407, error in (no error)=w1408) -> (queue out=w1405:refnum<queue>, error out=w1406:errorcluster)  [unwired: 1 in, 1 out]
          }
        }
      }
      frame "ERROR" {
        # "AN ERROR OCCURRED. STOP LOOP."
        n685 = call <vilib>:"Clear Errors.vi"("error in (no error)"=w1410) -> ("error out"=w1414:errorcluster)  [unwired: 5 in, 1 out]
      }
      frame "SHUTDOWN" {
        w1416 = FALSE ("FS-2012 ON|OFF")
        n686 = local write "POWER_SUPPLY ON|OFF 2"(w1416) -> ()
        n687 = local write "FS-2012 ON|OFF 2"(w1416) -> ()
        n688 = local write "ARDUINO ON|OFF 2"(w1416) -> ()
        n689 = Enqueue Element(queue=w1419, element="SHUTDOWN", error in (no error)=w1418) -> (queue out=w1421:refnum<queue>, error out=w1422:errorcluster)  [unwired: 1 in, 1 out]
      }
    }
    n690 = Wait Until Next ms Multiple(millisecond multiple=u32 20) -> ()  [unwired: 1 out]
  }
